vi "hostCommander_old2.vi"() -> ()   [LabVIEW 2014]
uses:
  <vilib>/Platform/TimedLoop/XDataNode/timing_clust.ctl
  <vilib>/Platform/TimedLoop/XDataNode/nitl_modes.ctl
  <vilib>/Platform/TimedLoop/XDataNode/wakeup.ctl
  <vilib>/dex/Stream Element Allocation Mode.ctl
  <vilib>/Analysis/1siggen.llb/Riffle Array (I32).vi
  <vilib>/platform/TimedLoop/XDataNode/XDataNode.xnode
  <resource>/objmgr/ni.dex.rc
  <vilib>/Platform/TimedLoop/XDataNode/XDNodeRunTimeDep.lvlib
  <vilib>/Analysis/NI_AALBase.lvlib
panel:
  out "Tab Control":enum32{"Host Commander"}(tab)
  out "reward#":i32=500
  in  "tickRate":u32=1
  in  "displayLength":dbl=10.0
  out "Digital Waveform Graph":digitalwaveform(graph)
  out "CurTrial#":u16
  out "stateMissed":bool
  out "VSmissed":bool
  out "VSbusy":bool=TRUE caption="VS"
  out "stateBusy":bool=TRUE caption="State"
  in  "FilePath":string="D:\\BehData\\"
  in  "FileName":string="debug"
  in  "Save data":bool=TRUE
  in  "Tab Control _2":T1(tab)
  in  "trialKey":i32[](array[numeric])
  in  "left":i32=300
  in  "right":i32=300
  in  "Initializeation Screen":dbl
  in  "Repeat":dbl
  in  "Interleave":bool
  in  "Randominze":bool
  in  "Blank":bool
  in  "Timing":sgl[](array[numeric])=[0.1, 0.2, 0.4, 0.6, 0.8, 1.0]
  in  "Orientation":sgl[](array[numeric])=[0.1, 0.2, 0.4, 0.6, 0.8, 1.0]
  in  "TF":sgl[](array[numeric])=[0.1, 0.2, 0.4, 0.6, 0.8, 1.0]
  in  "VS type":string="lick_reward"
  in  "SF":sgl[](array[numeric])=[0.04, 0.08, 0.16, 0.32, 0.45]
  in  "rtFIFOsize":u32=50
  in  "rtFIFOtimeout":u32
  in  "rtFIFOdataPool":u32=50
  in  "stateMachineCycle_uS":i64=500
  in  "vsFilterPeriod_uS":i32=500 format="%#1.6f"
  in  "lickThreshold_V":fxp<+/-,16,5>=1.0
  in  "vsThreshold_V":fxp<+/-,16,5>
  in  "audioThreshold_V":fxp<+/-,16,5>
  in  "audioFilterPeriod_uS":i32=50000 format="%#1.6f"
  in  "audioOffState_V":fxp<+/-,16,5>
  in  "manualShock":bool
  in  "manualWaterRight":bool
  in  "manualWaterLeft":bool
  in  "lickReward":bool
  in  "allowPunish":bool
  in  "beh type":string="ToneLickReward"
  in  "toneReward":bool=TRUE
  in  "rwdrefPeriod_uS":u32=500000
  in  "rewardPeriod_uS":u32=500000
  in  "waterOn_uS":u32=35000
  in  "timeout_uS":u32
  in  "shockOn_uS":u32
  in  "delay_uS":u32
  out "current state":u16(ring) items=["idle", "vs before", "vs", "vs after", "delay", "tone before", "tone", "tone after", "cycle end", "reward", "reward refractory", "punish", "punish refractory", "timeout", "exit"]
  out "Error 1":string
  out "Error 2":string
  out "Originating IP":string="192.168.137.2"
  out "Incoming data":string="TrlDone 1.000 "
  out "stream counter":u32
  out "Is Connected":bool
  out "Available Elements for Writing":i32
  in  "stream writer buffer size":i32=500
  in  "IP_VS":string="192.168.137.3"
  in  "IP_RT":string="192.168.137.2"
  in  "port_remote":u16=9091
  in  "IP_host":string="192.168.137.1"
  in  "port_local":u16=9090
  in  "IP_broadcast":string="192.168.137.255"
  out "INFO":string="Stop 1.000 "
  out "stop - local":bool=TRUE
  in  "Notes":string="14-4"
  in  "Abort":bool caption="run-stop"
  in  "run-stop":bool
  out "dispTimeout":bool
  out "saveTimeout":bool
  out "CurTrial# (remote)":u16
  in  "totalTrial#":u16=300
  out "CurTime (min)":i32
  in  "ITI_ms":i32=5000
  # "busy"
  # "missed"
  # "trialProbability"
  # "Errors for debugging"
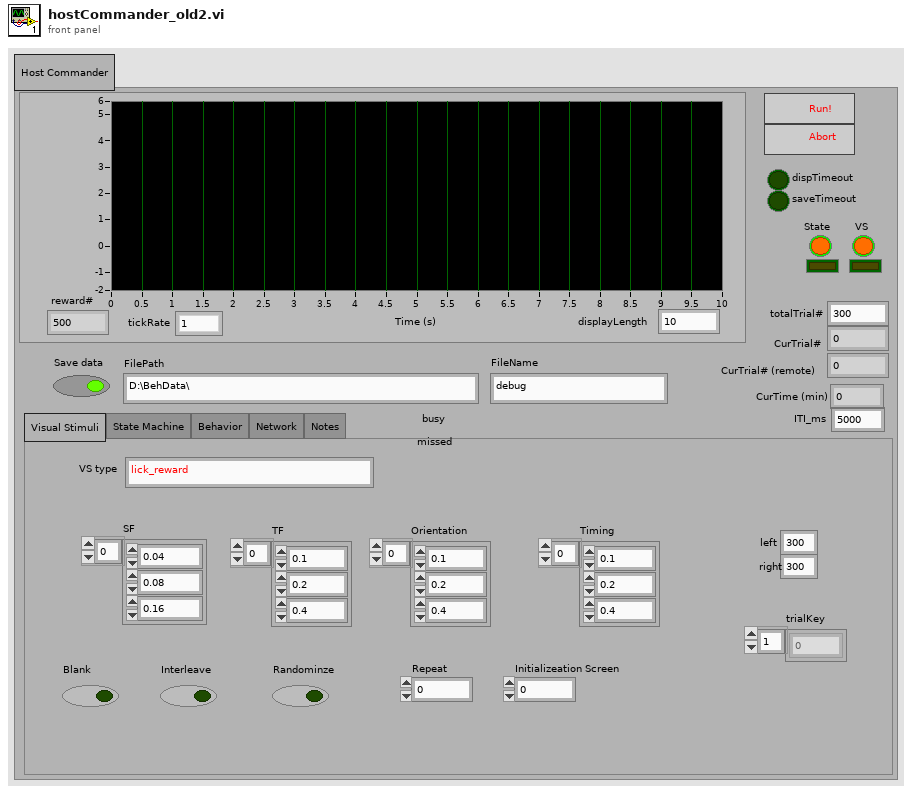
[diagram p1: front panel]
types:
  T1 = enum32{"Visual Stimuli", "State Machine", "Behavior", "Network", "Notes"}
  T2 = enum16{"open", "replace", "create", "open or create", "replace or create", "replace or create with confirmation"}
  T3 = enum16{"big-endian, network order", "native, host order", "little-endian"}
  T4 = typedef "XDNodeRunTimeDep.lvlib/timing_clust.ctl" = cluster{"Expected End [f-1]":u64, "Actual End [f-1]":u64, "Finished Late? [f-1]":bool, "Expected End [i-1]":u64, "Actual End [i-1]":u64, "Finished Late? [i-1]":bool, "Expected Start [i]":u64, "Actual Start [i]":u64, "Expected Start [f]":u64, "Actual Start [f]":u64, "Source Name":string, "Structure Name":string, "Period":i64, "Deadline":i64, "Offset":i64, "Start":i64, "Priority":i32, "Timeout":i32, "Mode":T5, "Wakeup Reason":T6, "Error":errorcluster, "Source Type":string, "Secondary Source Type":string, "Global End Time":u64, "Global Start Time":u64, "Frame Duration":u64, "Iteration Duration":u64, "Assigned CPU":i32, "I/O Scan Engine Mode":u32}
  T5 = typedef "XDNodeRunTimeDep.lvlib/nitl_modes.ctl" = enum32{"No Change", "Process missed periods, maintain original phase", "Discard missed periods, maintain original phase", "Process missed periods, ignore original phase", "Discard missed periods, ignore original phase"}
  T6 = typedef "XDNodeRunTimeDep.lvlib/wakeup.ctl" = enum32{"Normal", "Aborted", "Asynchronous wakeup", "Timing source error", "Timed loop error", "Timeout"}
  T7 = typedef "Stream Element Allocation Mode.ctl" = u32
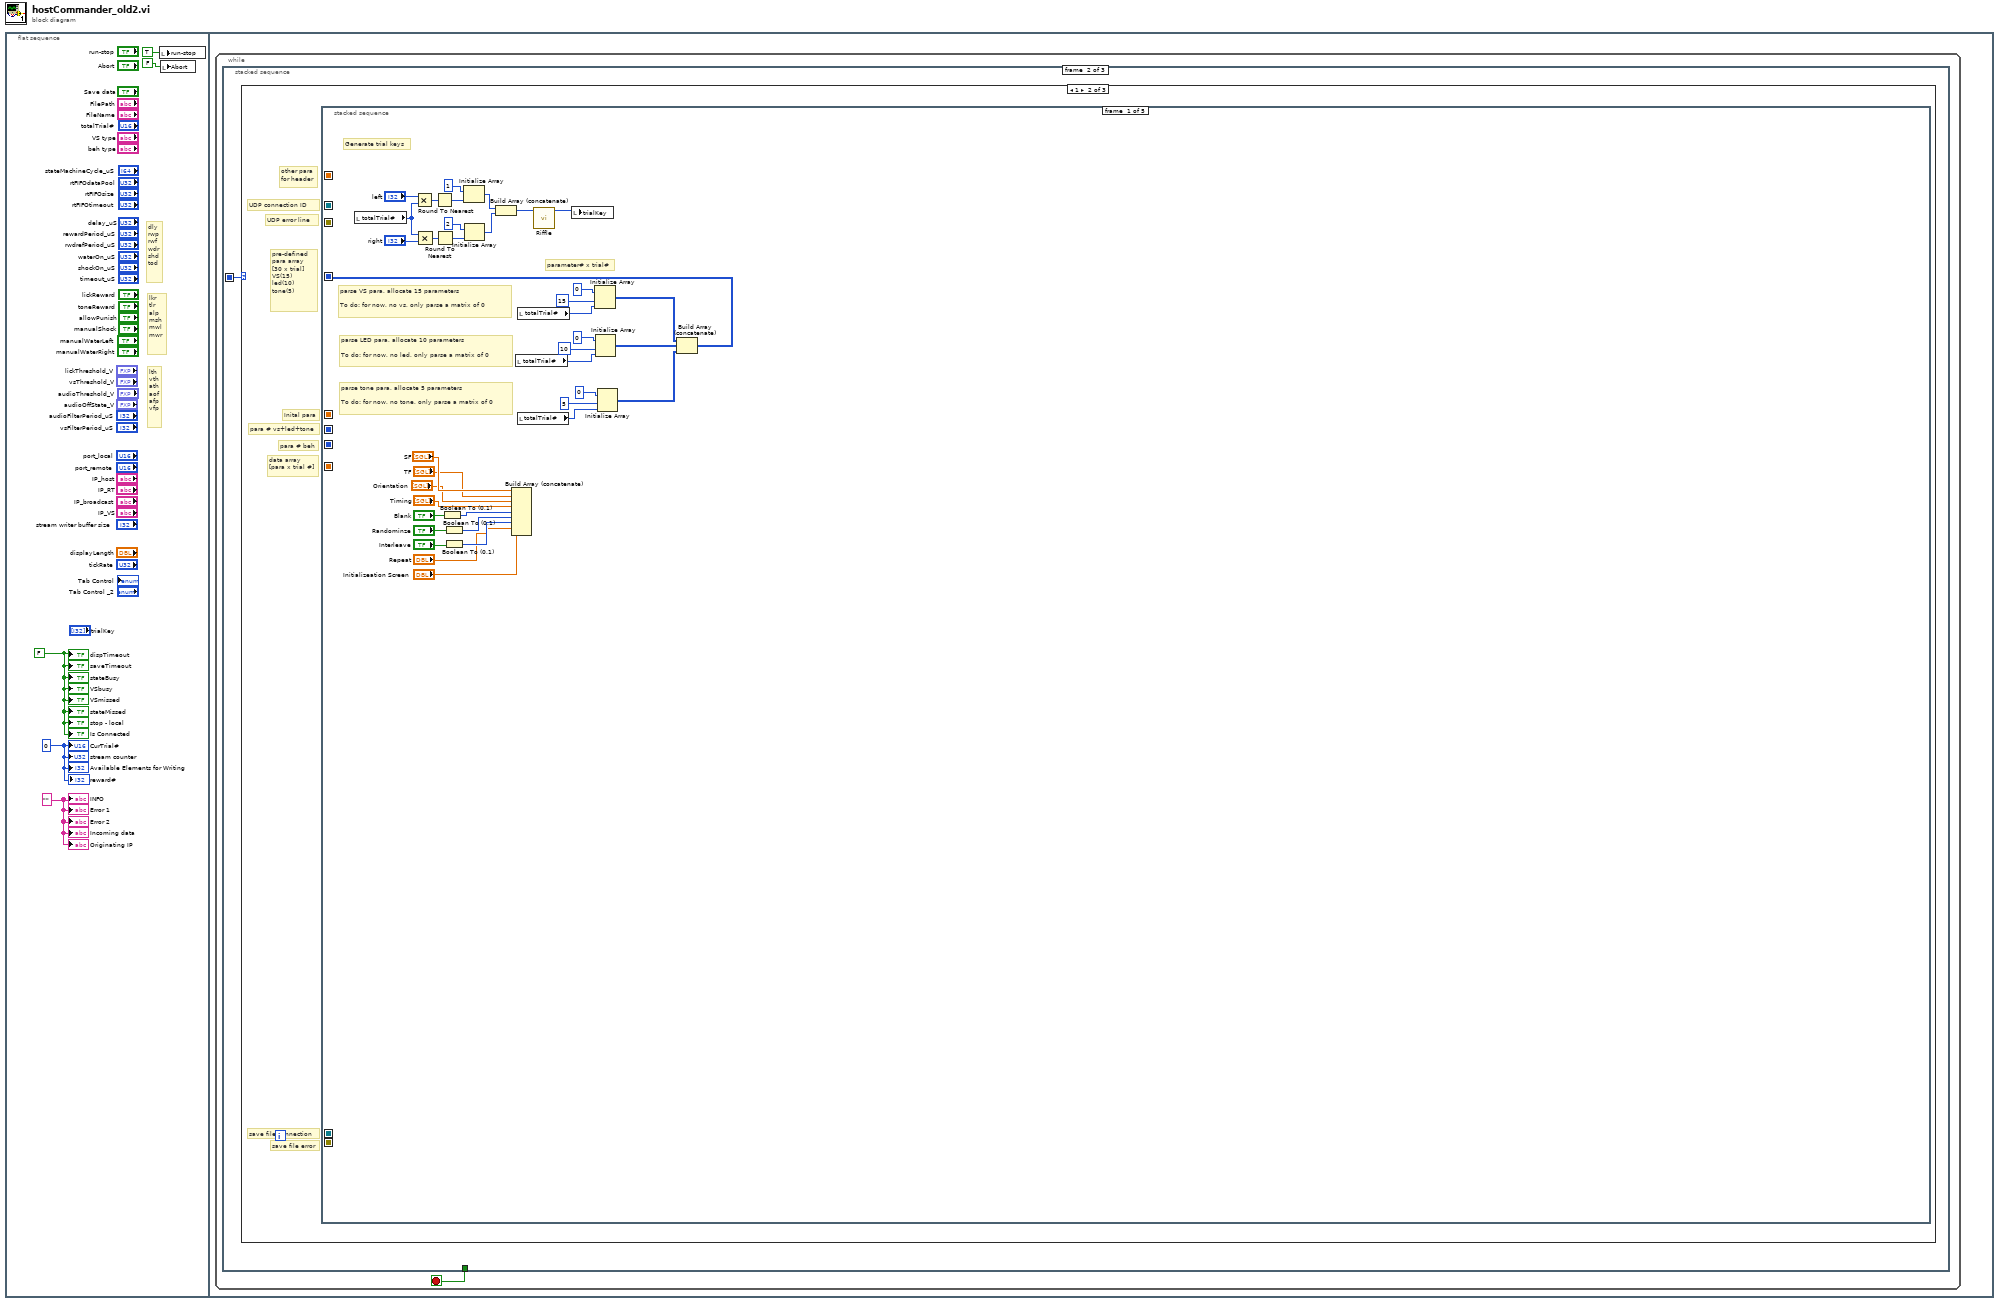
[diagram p0: block diagram]
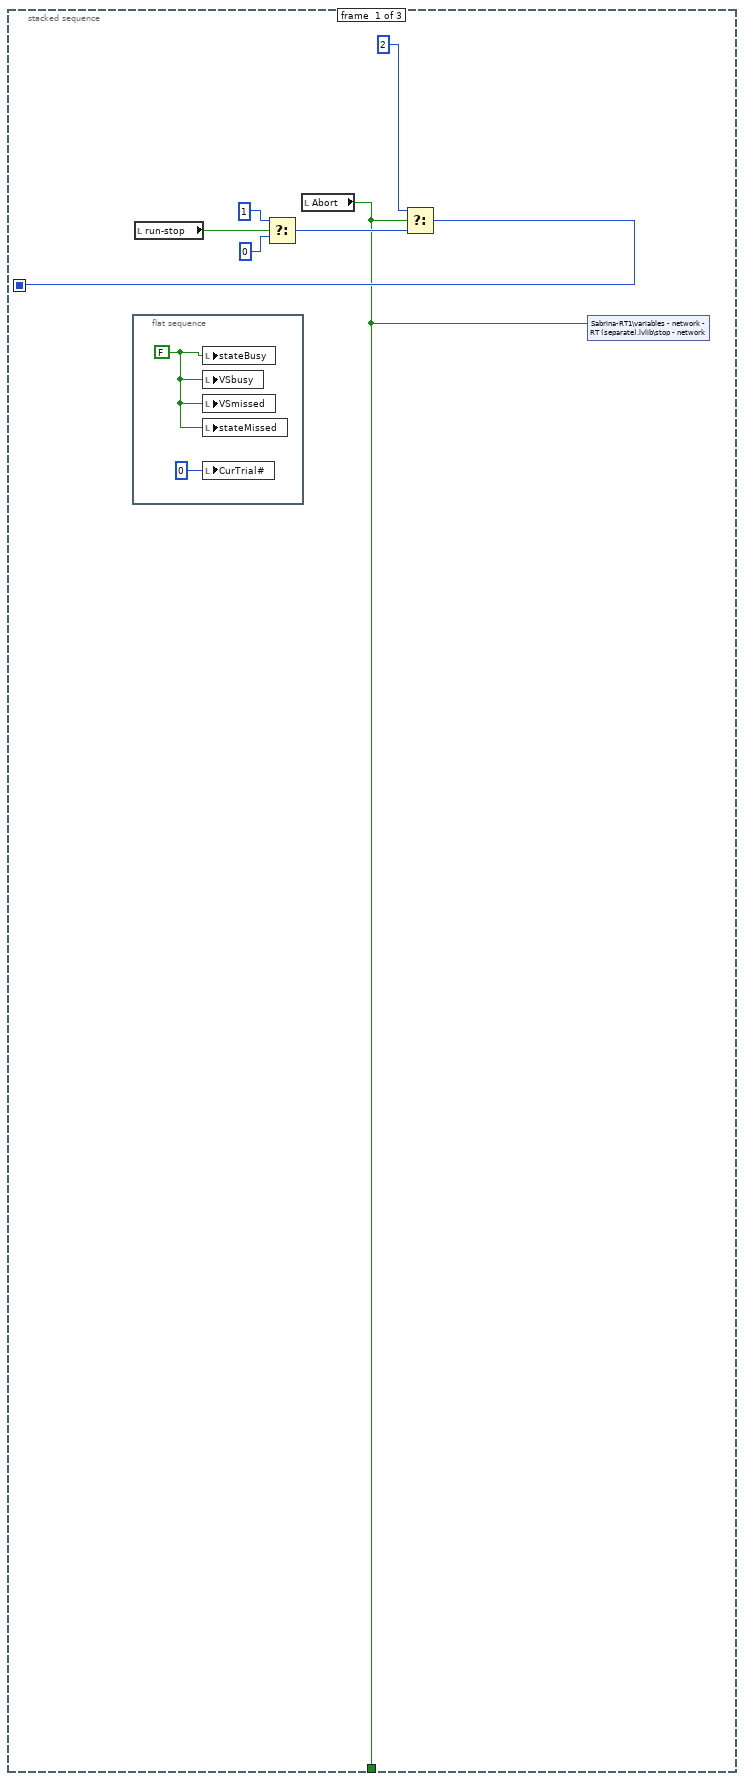
[diagram p2: hidden frame]
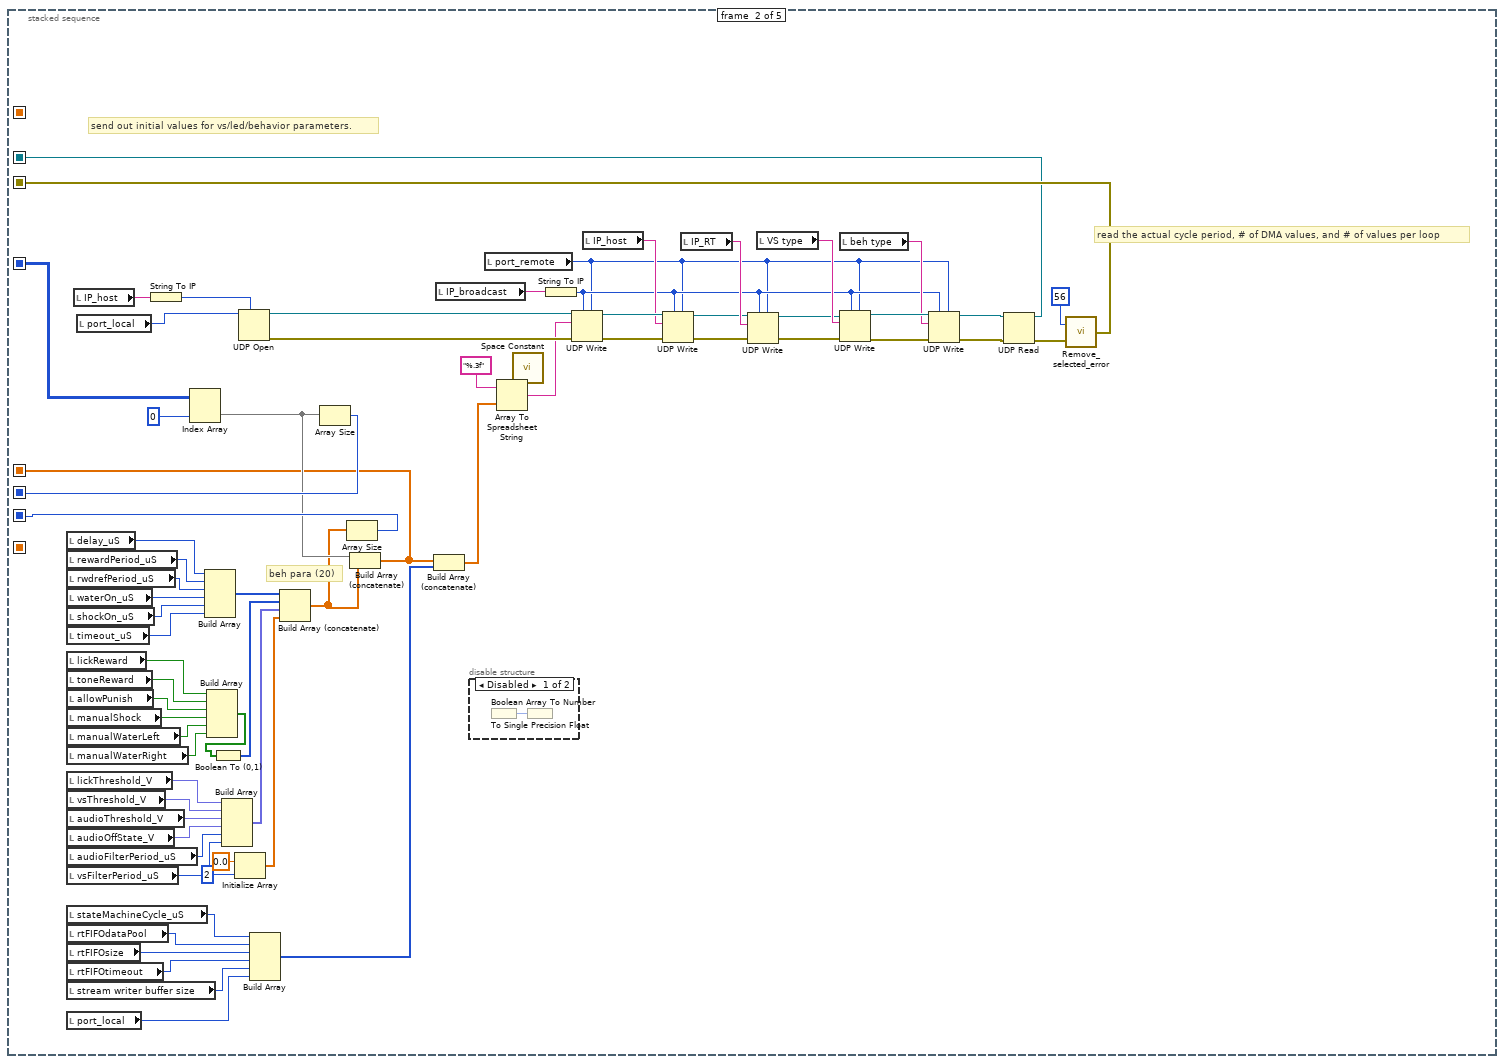
[diagram p4: hidden frame]
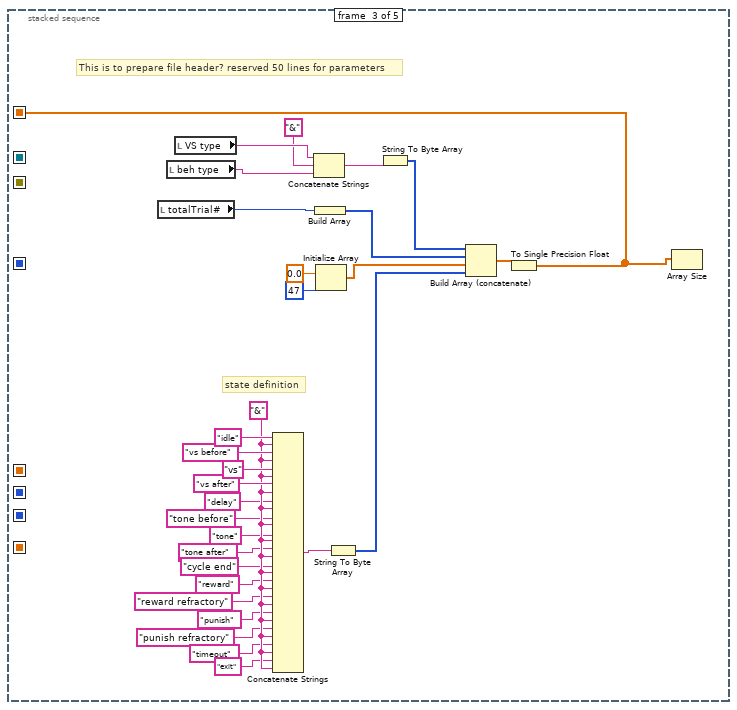
[diagram p6: hidden frame]
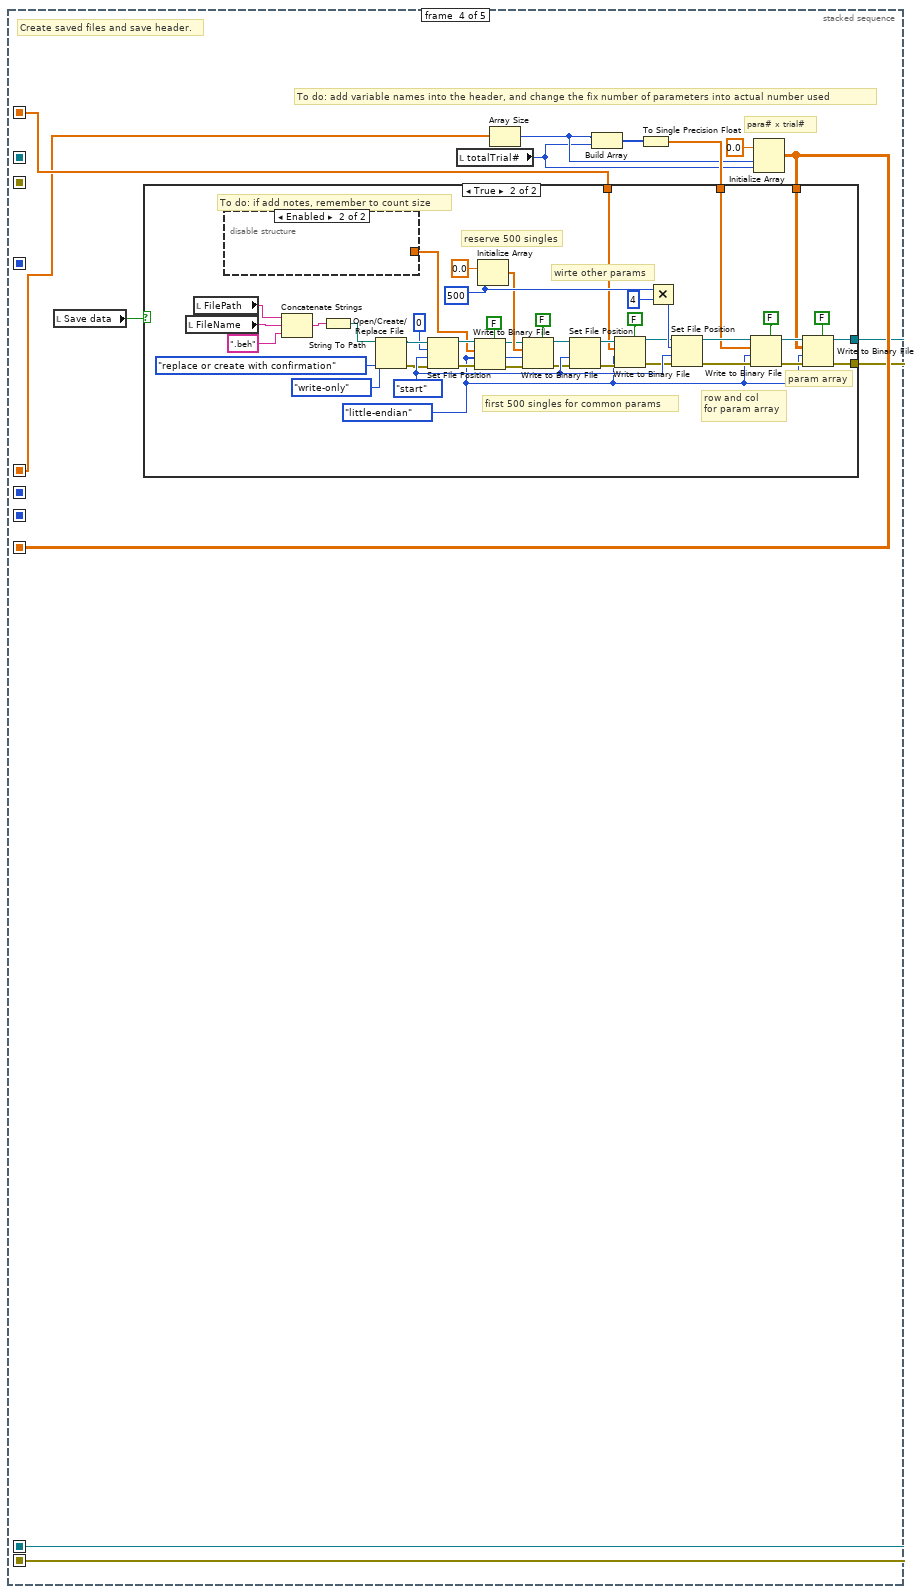
[diagram p7: hidden frame]
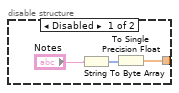
[diagram p9: hidden frame]
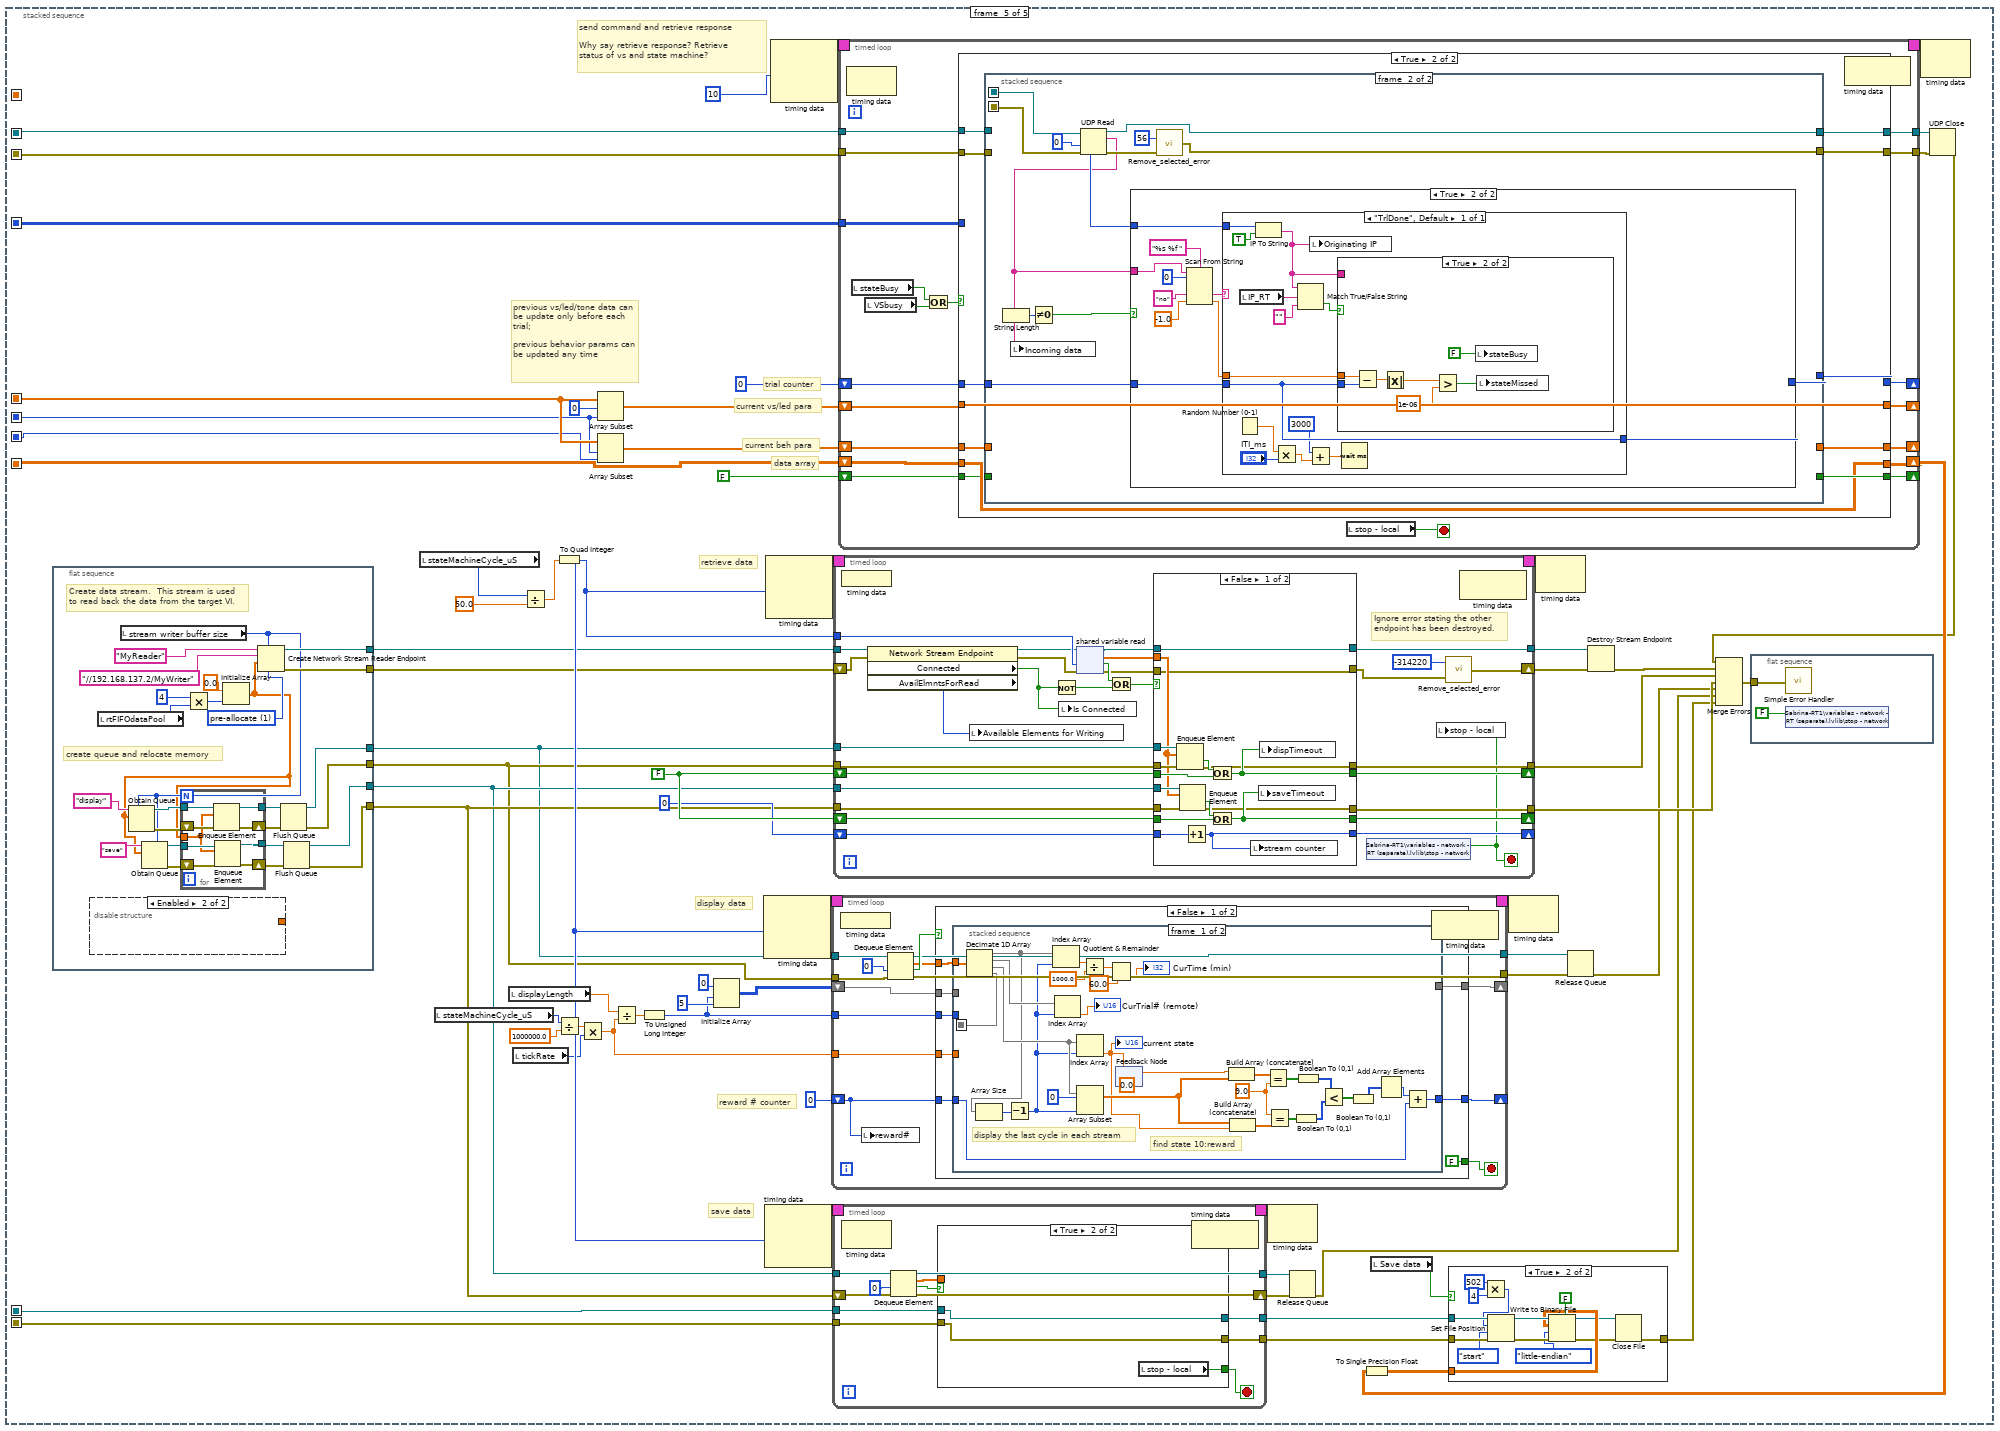
[diagram p10: hidden frame]
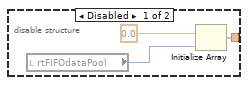
[diagram p11: hidden frame]
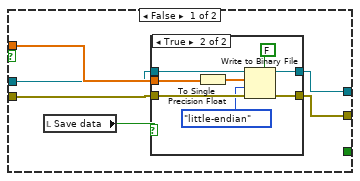
[diagram p12: hidden frame]
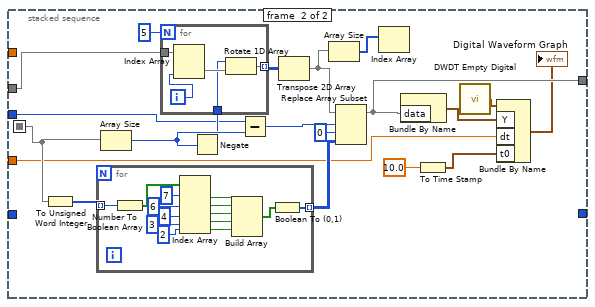
[diagram p14: hidden frame]
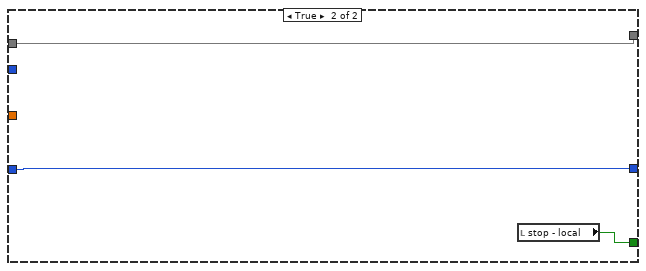
[diagram p15: hidden frame]
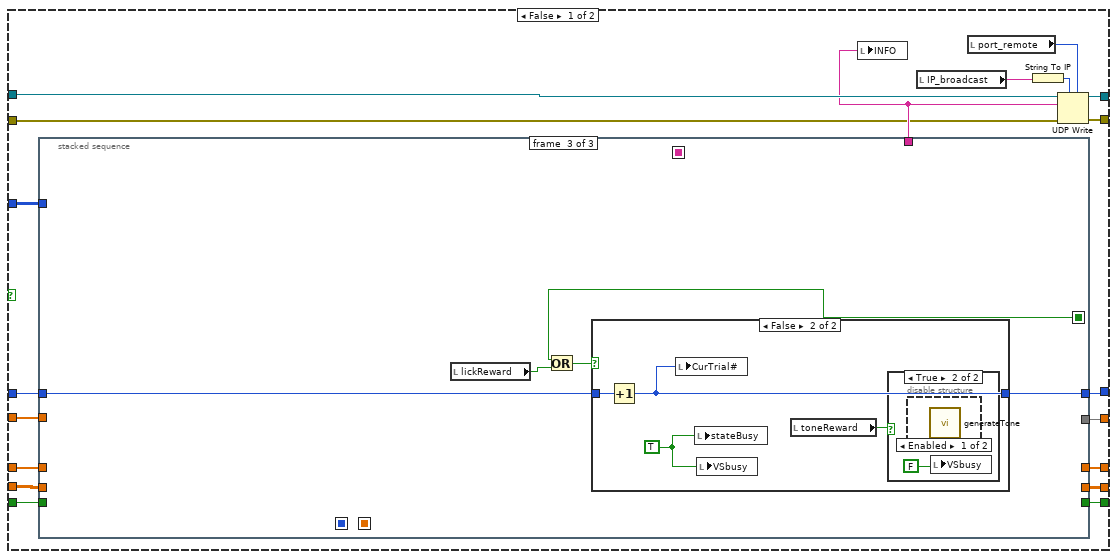
[diagram p17: hidden frame]
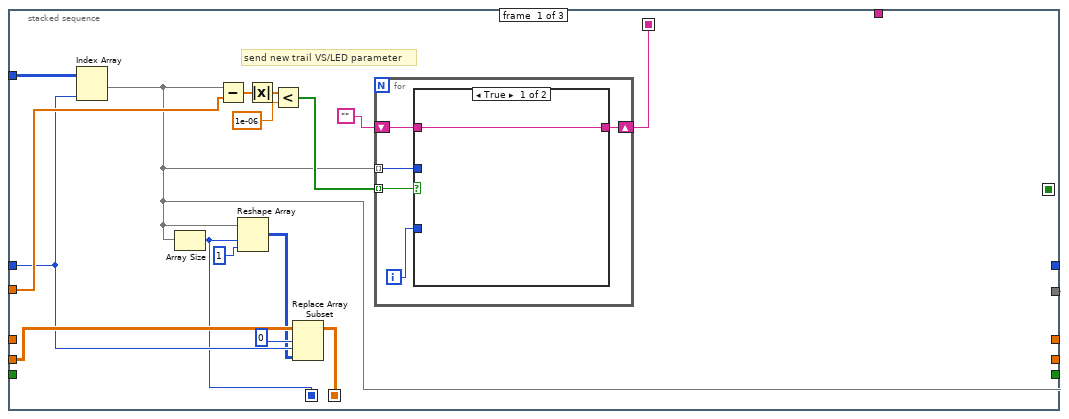
[diagram p18: hidden frame]
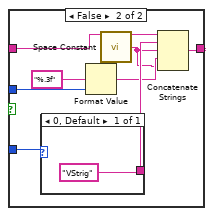
[diagram p19: hidden frame]
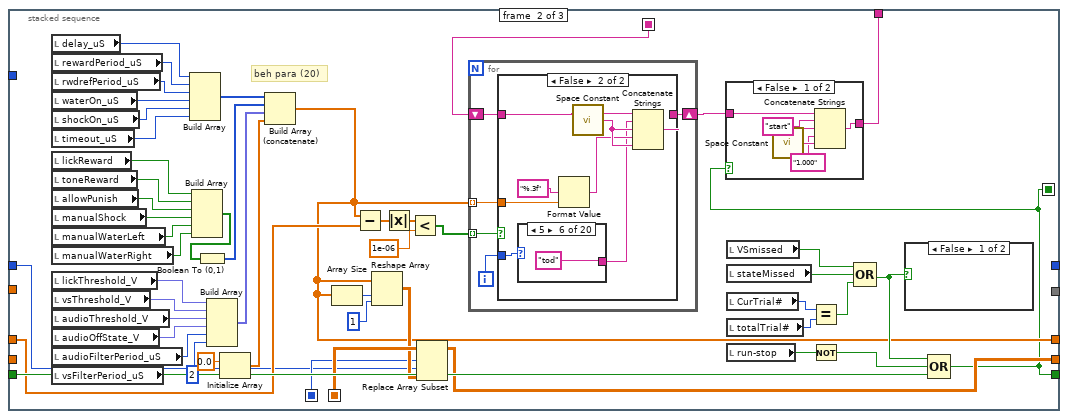
[diagram p20: hidden frame]
diagram:
  n1 = flat-sequence {
    frame #0 {
      w2 = ""
      w1 = 0
      w3 = FALSE
      # "lth\nvth\nath\naof\nafp\nvfp"
      # "dly\nrwp\nrwf\nwdr\nshd\ntod"
      # "lkr\ntlr\nalp\nmsh\nmwl\nmwr"
      n2 = local write "run-stop"(TRUE) -> ()
      n3 = local write "Abort"(FALSE) -> ()
      "dispTimeout" <- w3
      "saveTimeout" <- w3
      "stateBusy" <- w3
      "VSbusy" <- w3
      "VSmissed" <- w3
      "stateMissed" <- w3
      "CurTrial#" <- w1
      "stop - local" <- w3
      "INFO" <- w2
      "Error 2" <- w2
      "Error 1" <- w2
      "Available Elements for Writing" <- w1
      "Is Connected" <- w3
      "stream counter" <- w1
      "Incoming data" <- w2
      "Originating IP" <- w2
      "reward#" <- w1
    }
    frame #1 {
      n4 = while {
        stop <- w6 stop-if-true
        n5 = stacked-sequence {
          seq-local: [w8 _ _] -> [_ w16 _]
          tunnel: [w7 _ _] -> w6
          frame #0 {
            n6 = flat-sequence {
              frame #0 {
                w15 = FALSE
                n7 = local write "stateBusy"(w15) -> ()
                n8 = local write "VSbusy"(w15) -> ()
                n9 = local write "VSmissed"(w15) -> ()
                n10 = local write "stateMissed"(w15) -> ()
                n11 = local write "CurTrial#"(0) -> ()
              }
            }
            n12 = local read "run-stop"() -> (w10:bool)
            n13 = Select(t=u8 1, s=w10, f=u8 0) -> (s? t:f=w9:u8)
            n14 = local read "Abort"() -> (w7:bool)
            n15 = Select(t=u8 2, s=w7, f=w9) -> (s? t:f=w8:u8)
            n16 = shared-variable "Sabrina-RT1\\variables - network - RT (separate).lvlib\\stop - network"(w7) -> ()  [unwired: 1 in, 1 out]
          }
          frame #1 {
            n17 = case shown="1" w16 {
              frame 0, Default {
              }
              frame 1 {
                # "para # beh"
                # "save file error"
                # "save file connection"
                # "data array\n[para x trial #]"
                # "other para\nfor header"
                # "UDP error line"
                # "UDP connection ID"
                # "para # vs+led+tone"
                # "Inital para"
                # "pre-defined \npara array\n[30 x trial]\nVS(15)\nled(10)\ntone(5)"
                n18 = stacked-sequence {
                  seq-local: [_ w105 _ _ _] -> [_ _ _ _ w264]
                  seq-local: [_ w102 _ _ _] -> [_ _ _ _ w265]
                  seq-local: [_ w55 _ _ _] -> [_ _ _ w157 w263]
                  seq-local: [_ w69 _ _ _] -> [_ _ _ _ w213]
                  seq-local: [w37 _ _ _ _] -> [_ w106 _ _ w256]
                  seq-local: [_ _ w125 _ _] -> [_ _ _ w161 _]
                  seq-local: [_ _ _ w160 _] -> [_ _ _ _ w255]
                  seq-local: [_ _ _ w159 _] -> [_ _ _ _ w235]
                  seq-local: [_ _ _ w158 _] -> [_ _ _ _ w236]
                  seq-local: [_ w70 _ _ _] -> [_ _ _ _ w215]
                  frame #0 {
                    # "parameter# x trial#"
                    # "parse tone para, allocate 5 parameters \n\nTo do: for now, no tone, only parse a matrix of 0"
                    # "parse LED para, allocate 10 parameters \n\nTo do: for now, no led, only parse a matrix of 0"
                    # "parse VS para, allocate 15 parameters \n\nTo do: for now, no vs, only parse a matrix of 0"
                    # "Generate trial keys"
                    n19 = local read "totalTrial#"() -> (w21:u16)
                    n20 = Multiply(x="left", y=w21) -> (x*y=w28:i32)
                    n21 = Multiply(x=w21, y="right") -> (x*y=w23:i32)
                    n22 = Round To Nearest(number=w28) -> (nearest integer value=w26:i32)
                    n23 = Round To Nearest(number=w23) -> (nearest integer value=w25:i32)
                    n24 = Boolean To (0,1)(Boolean="Blank") -> (0, 1=w49:i16)
                    n25 = Boolean To (0,1)(Boolean="Interleave") -> (0, 1=w44:i16)
                    n26 = Boolean To (0,1)(Boolean="Randominze") -> (0, 1=w48:i16)
                    n27 = Initialize Array(1, w26) -> (w20:i32[])
                    n28 = Initialize Array(2, w25) -> (w19:i32[])
                    n29 = Build Array (concatenate)(w20, w19) -> (w18:i32[])
                    n30 = Build Array (concatenate)("SF", "TF", "Orientation", "Timing", w49, w48, w44, "Repeat", "Initializeation Screen") -> ()  [unwired: 1 out]
                    n31 = local read "totalTrial#"() -> (w35:u16)
                    n32 = local read "totalTrial#"() -> (w34:u16)
                    n33 = local read "totalTrial#"() -> (w36:u16)
                    n34 = call-poly <vilib>:"Riffle.vi"("X"=w18) -> ("Riffled {X}"=w17:i32[])  [unwired: 8 in, 2 out]
                    n35 = local write "trialKey"(w17) -> ()
                    n36 = Initialize Array(0, 15, w36) -> (w40:i32[][])
                    n37 = Initialize Array(0, 10, w35) -> (w39:i32[][])
                    n38 = Initialize Array(0, 5, w34) -> (w38:i32[][])
                    n39 = Build Array (concatenate)(w40, w39, w38) -> (w37:i32[][])
                  }
                  frame #1 {
                    # "beh para (20)"
                    # "read the actual cycle period, # of DMA values, and # of values per loop"
                    # "send out initial values for vs/led/behavior parameters."
                    n40 = local read "delay_uS"() -> (w99:u32)
                    n41 = local read "rewardPeriod_uS"() -> (w98:u32)
                    n42 = local read "rwdrefPeriod_uS"() -> (w97:u32)
                    n43 = local read "waterOn_uS"() -> (w96:u32)
                    n44 = local read "shockOn_uS"() -> (w95:u32)
                    n45 = local read "timeout_uS"() -> (w94:u32)
                    n46 = local read "lickReward"() -> (w93:bool)
                    n47 = local read "toneReward"() -> (w92:bool)
                    n48 = local read "allowPunish"() -> (w91:bool)
                    n49 = local read "manualShock"() -> (w90:bool)
                    n50 = local read "manualWaterLeft"() -> (w89:bool)
                    n51 = local read "manualWaterRight"() -> (w88:bool)
                    n52 = local read "lickThreshold_V"() -> (w87:fxp<+/-,16,5>)
                    n53 = local read "vsThreshold_V"() -> (w86:fxp<+/-,16,5>)
                    n54 = local read "audioThreshold_V"() -> (w85:fxp<+/-,16,5>)
                    n55 = local read "audioOffState_V"() -> (w82:fxp<+/-,16,5>)
                    n56 = local read "audioFilterPeriod_uS"() -> (w84:i32)
                    n57 = local read "vsFilterPeriod_uS"() -> (w83:i32)
                    n58 = local read "stateMachineCycle_uS"() -> (w81:i64)
                    n59 = local read "rtFIFOdataPool"() -> (w79:u32)
                    n60 = local read "rtFIFOsize"() -> (w78:u32)
                    n61 = local read "rtFIFOtimeout"() -> (w80:u32)
                    n62 = local read "stream writer buffer size"() -> (w77:i32)
                    n63 = local read "port_local"() -> (w68:u16)
                    n64 = local read "IP_host"() -> (w120:string)
                    n65 = local read "port_local"() -> (w118:u16)
                    n66 = String To IP(1:w120) -> (0:w119:u32)
                    n67 = Index Array(array=w106, index (col)=0) -> (element=w57:i32[])  [unwired: 1 in]
                    n68 = Build Array(w99, w98, w97, w96, w95, w94) -> (w76:u32[])
                    n69 = Build Array(w93, w92, w91, w90, w89, w88) -> (w59:bool[])
                    n70 = Boolean To (0,1)(Boolean=w59) -> (0, 1=w58:i16[])
                    n71 = Build Array(w87, w86, w85, w82, w84, w83) -> (w75:fxp<+/-,43,32>[])
                    n72 = Initialize Array(sgl 0.0, 2) -> (w71:sgl[])
                    n73 = UDP Open(7:w119, 11:w118) -> (port=w116:refnum<k16>, 0:w117:errorcluster)  [unwired: 3 in, 1 out]
                    n74 = Build Array(w81, w79, w78, w80, w77, w68) -> (w74:i64[])
                    n75 = Build Array (concatenate)(w76, w58, w75, w71) -> (w56:sgl[])
                    n76 = Array Size(array=w57) -> (size(s)=w69:i32)
                    n77 = Array Size(array=w56) -> (size(s)=w70:i32)
                    n78 = Build Array (concatenate)(w57, w56) -> (w55:sgl[])
                    n79 = Build Array (concatenate)(w55, w74) -> (w107:sgl[])
                    n80 = local read "IP_broadcast"() -> (w121:string)
                    n81 = disable-structure shown="Disabled" {
                      frame Disabled {
                        n82 = Boolean Array To Number() -> (number=w122:u32)  [unwired: 1 in]
                        n83 = To Single Precision Float(number=w122) -> ()  [unwired: 1 out]
                      }
                      frame Enabled {
                      }
                    }
                    n84 = local read "port_remote"() -> (w63:u16)
                    n85 = call <vilib>:"Space Constant.vi"() -> ("String"=w109:string)
                    n86 = Array To Spreadsheet String ("beh para")(delimiter (Tab)=w109, array=w107, 3:"%.3f" ("format string")) -> (spreadsheet string=w108:string)
                    n87 = String To IP(1:w121) -> (0:w64:u32)
                    n88 = UDP Write(address=w64, port or service name=w63, connection ID=w116, data in=w108, 8:w117) -> (error out=w115:errorcluster, 3:w67:refnum<k16>)  [unwired: 1 in]
                    n89 = local read "IP_host"() -> (w66:string)
                    n90 = UDP Write(address=w64, port or service name=w63, connection ID=w67, data in=w66) -> (3:w62:refnum<k16>)  [unwired: 2 in, 1 out]
                    n91 = local read "IP_RT"() -> (w65:string)
                    n92 = UDP Write(address=w64, port or service name=w63, connection ID=w62, data in=w65) -> (3:w61:refnum<k16>)  [unwired: 2 in, 1 out]
                    n93 = local read "VS type"() -> (w114:string)
                    n94 = local read "beh type"() -> (w111:string)
                    n95 = UDP Write(address=w64, port or service name=w63, connection ID=w61, data in=w114, 8:w115) -> (error out=w113:errorcluster, 3:w112:refnum<k16>)  [unwired: 1 in]
                    n96 = UDP Write(address=w64, port or service name=w63, connection ID=w112, data in=w111, 8:w113) -> (error out=w103:errorcluster, 3:w104:refnum<k16>)  [unwired: 1 in]
                    n97 = UDP Read(connection ID=w104, 8:w103) -> (error out=w101:errorcluster, 3:w102:refnum<k16>)  [unwired: 2 in, 3 out]
                    n98 = call "Remove_selected_error.vi"("error in (no error)"=w101, "errorCode"=56) -> ("error out"=w105:errorcluster)
                  }
                  frame #2 {
                    w137 = "&" ("string")
                    # "state definition"
                    # "This is to prepare file header? reserved 50 lines for parameters"
                    n99 = local read "totalTrial#"() -> (w145:u16)
                    n100 = local read "beh type"() -> (w123:string)
                    n101 = local read "VS type"() -> (w140:string)
                    n102 = Concatenate Strings("idle", w137, "vs before", w137, "vs", w137, "vs after", w137, "delay", w137, "tone before", w137, "tone", w137, "tone after", w137, "cycle end", w137, "reward", w137, "reward refractory", w137, "punish", w137, "punish refractory", w137, "timeout", w137, "exit", w137) -> (w150:string)
                    n103 = Concatenate Strings(w140, "&" ("string"), w123) -> (w139:string)
                    n104 = Build Array(w145) -> (w144:u16[])
                    n105 = Initialize Array(sgl 0.0 ("element"), 47 ("dimension size")) -> (w143:sgl[])
                    n106 = String To Byte Array(string=w150) -> (unsigned byte array=w142:u8[])
                    n107 = String To Byte Array(string=w139) -> (unsigned byte array=w138:u8[])
                    n108 = Build Array (concatenate)(w138, w144, w143, w142) -> (w141:sgl[])
                    n109 = To Single Precision Float(number=w141) -> (single precision float=w125:sgl[])
                    n110 = Array Size(array=w125) -> ()  [unwired: 1 out]
                  }
                  frame #3 {
                    # "To do: add variable names into the header, and change the fix number of parameters into actual number used"
                    # "para# x trial#"
                    # "Create saved files and save header."
                    n111 = local read "Save data"() -> (w163:bool)
                    n112 = local read "totalTrial#"() -> (w153:u16)
                    n113 = Array Size(array=w157) -> (size(s)=w154:i32)
                    n114 = Build Array(w154, w153) -> (w156:i32[])
                    n115 = To Single Precision Float(number=w156) -> (single precision float=w155:sgl[])
                    n116 = Initialize Array(sgl 0.0 ("element"), w154, w153) -> (w160:sgl[][])
                    n117 = case shown="True" w163 {
                      tunnel: w155 -> [_ w180]
                      tunnel: w161 -> [_ w164]
                      tunnel: w160 -> [_ w179]
                      tunnel: [_ w177] -> w158
                      tunnel: [_ w178] -> w159
                      frame False {
                      }
                      frame True {
                        w198 = 500 ("dimension size")
                        w171 = T3."little-endian" ("byte order (0:big-endian, network order)")
                        w199 = enum16{"start", "end", "current"}."start" ("from (0:start)")
                        # "To do: if add notes, remember to count size"
                        # "param array"
                        # "row and col\nfor param array"
                        # "first 500 singles for common params"
                        # "reserve 500 singles"
                        # "wirte other params"
                        n118 = local read "FileName"() -> (w166:string)
                        n119 = local read "FilePath"() -> (w169:string)
                        n120 = disable-structure shown="Enabled" {
                          disable-tunnel: [w206 _] -> w170
                          frame Disabled {
                            n121 = String To Byte Array(string="Notes") -> (unsigned byte array=w207:u8[])
                            n122 = To Single Precision Float(number=w207) -> (single precision float=w206:sgl[])
                          }
                          frame Enabled {
                          }
                        }
                        n123 = Concatenate Strings(w169, w166, ".beh" ("string")) -> (w168:string)
                        n124 = String To Path(string=w168) -> (path=w167:path)
                        n125 = Open/Create/Replace File(file path (use dialog)=w167, operation (0:open)=T2."replace or create with confirmation", access (0:read/write)=enum16{"read/write", "read-only", "write-only"}."write-only") -> (refnum out=w184:refnum<file>, error out=w185:errorcluster)  [unwired: 3 in, 1 out]
                        n126 = Set File Position(offset (in bytes) (0)=i64 0, refnum=w184, from (0:start)=w199, error in=w185) -> (refnum out=w175:refnum<file>, error out=w173:errorcluster)
                        n127 = Write to Binary File(file (use dialog)=w175, data=w170, error in=w173, 5:FALSE ("prepend array or string size? (T)"), 9:w171) -> (refnum out=w174:refnum<file>, error out=w172:errorcluster)  [unwired: 1 in, 1 out]
                        n128 = Initialize Array(sgl 0.0 ("element"), w198) -> (w188:sgl[])
                        n129 = Write to Binary File(file (use dialog)=w174, data=w188, error in=w172, 5:FALSE ("prepend array or string size? (T)"), 9:w171) -> (refnum out=w190:refnum<file>, error out=w191:errorcluster)  [unwired: 1 in, 1 out]
                        n130 = Set File Position(refnum=w190, from (0:start)=w199, error in=w191) -> (refnum out=w192:refnum<file>, error out=w193:errorcluster)  [unwired: 1 in]
                        n131 = Write to Binary File(file (use dialog)=w192, data=w164, error in=w193, 5:FALSE ("prepend array or string size? (T)"), 9:w171) -> (refnum out=w194:refnum<file>, error out=w195:errorcluster)  [unwired: 1 in, 1 out]
                        n132 = Multiply(x=w198, y=4) -> (x*y=w196:i32)
                        n133 = Set File Position(offset (in bytes) (0)=w196, refnum=w194, from (0:start)=w199, error in=w195) -> (refnum out=w201:refnum<file>, error out=w202:errorcluster)
                        n134 = Write to Binary File(file (use dialog)=w201, data=w180, error in=w202, 5:FALSE ("prepend array or string size? (T)"), 9:w171) -> (refnum out=w203:refnum<file>, error out=w204:errorcluster)  [unwired: 1 in, 1 out]
                        n135 = Write to Binary File(file (use dialog)=w203, data=w179, error in=w204, 5:FALSE ("prepend array or string size? (T)"), 9:w171) -> (refnum out=w177:refnum<file>, error out=w178:errorcluster)  [unwired: 1 in, 1 out]
                      }
                    }
                  }
                  frame #4 {
                    w270 = FALSE
                    # "reward # counter"
                    # "save data"
                    # "data array"
                    # "current beh para"
                    # "current vs/led para"
                    # "trial counter"
                    # "previous vs/led/tone data can be update only before each trial;\n\nprevious behavior params can be updated any time"
                    # "display data"
                    # "retrieve data"
                    # "send command and retrieve response\n\nWhy say retrieve response? Retrieve\nstatus of vs and state machine?"
                    n136 = flat-sequence {
                      tunnel: [w297] -> w221
                      tunnel: [w296] -> w220
                      tunnel: [w285] -> w219
                      tunnel: [w284] -> w218
                      tunnel: [w283] -> w217
                      tunnel: [w282] -> w216
                      frame #0 {
                        w299 = T7 1 items=["allocate as needed", "pre-allocate"] ("element allocation mode")
                        # "create queue and relocate memory"
                        # "Create data stream.  This stream is used\nto read back the data from the target VI."
                        n137 = disable-structure shown="Enabled" {
                          disable-tunnel: [w302 _] -> _
                          frame Disabled {
                            n138 = local read "rtFIFOdataPool"() -> (w303:u32)
                            n139 = Initialize Array(sgl 0.0, w303) -> (w302:sgl[])
                          }
                          frame Enabled {
                          }
                        }
                        n140 = local read "rtFIFOdataPool"() -> (w278:u32)
                        n141 = local read "stream writer buffer size"() -> (w281:i32)
                        n142 = Multiply(x=4, y=w278) -> (x*y=w277:u32)
                        n143 = Initialize Array(sgl 0.0, w277) -> (w280:sgl[])
                        n144 = Obtain Queue(max queue size (-1, unlimited)=w281, name (unnamed)="display", element data type=w280) -> (queue out=w288:refnum<queue>, error out=w289:errorcluster)  [unwired: 2 in, 1 out]
                        n145 = Obtain Queue(max queue size (-1, unlimited)=w281, name (unnamed)="save", element data type=w280) -> (queue out=w290:refnum<queue>, error out=w291:errorcluster)  [unwired: 2 in, 1 out]
                        n146 = for {
                          N: w281 -> [_]
                          tunnel: w288 -> [w313]
                          tunnel: [w312] -> w294
                          shift-right: [w310] -> w295
                          shift-left: w289 -> [w311]
                          shift-right: [w306] -> w293
                          shift-left: w291 -> [w307]
                          tunnel: w290 -> [w309]
                          tunnel: [w308] -> w292
                          tunnel: w280 -> [w305]
                          n147 = Enqueue Element(queue=w313, element=w305, error in (no error)=w311) -> (queue out=w312:refnum<queue>, error out=w310:errorcluster)  [unwired: 1 in, 1 out]
                          n148 = Enqueue Element(queue=w309, element=w305, error in (no error)=w307) -> (queue out=w308:refnum<queue>, error out=w306:errorcluster)  [unwired: 1 in, 1 out]
                        }
                        n149 = Create Network Stream Reader Endpoint(6:w299, 7:w281, 9:w280, 10:"//192.168.137.2/MyWriter" ("reader name"), 11:"MyReader" ("reader name")) -> (0:w297:errorcluster, 3:w296:refnum<k21>)  [unwired: 2 in]
                        n150 = Flush Queue(queue=w294, error in (no error)=w295) -> (queue out=w282:refnum<queue>, error out=w283:errorcluster)  [unwired: 1 out]
                        n151 = Flush Queue(queue=w292, error in (no error)=w293) -> (queue out=w284:refnum<queue>, error out=w285:errorcluster)  [unwired: 1 out]
                      }
                    }
                    n152 = local read "stateMachineCycle_uS"() -> (w273:i64)
                    n153 = local read "stateMachineCycle_uS"() -> (w249:i64)
                    n154 = local read "displayLength"() -> (w243:dbl)
                    n155 = local read "tickRate"() -> (w211:u32)
                    n156 = Divide(x=w273, y=sgl 50.0) -> (x/y=w272:sgl)
                    n157 = To Quad Integer(1:w272) -> (0:w222:i64)
                    n158 = Divide(x=w249, y=1000000.0) -> (x/y=w212:dbl)
                    n159 = Multiply(x=w212, y=w211) -> (x*y=w210:dbl)
                    n160 = Array Subset(array=w263, index=0, length=w213) -> (w261:sgl[])
                    n161 = Array Subset(array=w263, index=w213, length=w215) -> (w262:sgl[])
                    n162 = Divide(x=w243, y=w210) -> (x/y=w246:dbl)
                    n163 = To Unsigned Long Integer(number=w246) -> (unsigned 32bit integer=w244:u32)
                    n164 = Initialize Array(u8 0, w244, 5 ("dimension size")) -> (w245:u8[][])
                    n165 = node-c288(w222) -> (w242:T4)  [unwired: 2 in]
                    n166 = node-c288(w222) -> (w240:T4)  [unwired: 2 in]
                    n167 = node-c288(w222) -> (w276:T4)  [unwired: 2 in]
                    n168 = node-c288(10) -> (w267:T4)  [unwired: 2 in]
                    n169 = timed-loop {
                      tunnel: w216 -> [w366]
                      tunnel: w217 -> [w365]
                      shift-right: [w362] -> _
                      shift-left: u32 0 -> [w353]
                      shift-right: [w359] -> _
                      shift-left: w245 -> [w361]
                      tunnel: w244 -> [w360]
                      timing: w242 -> [_]
                      timing-out: [_] -> w241
                      tunnel: [w356] -> w232
                      tunnel: [w355] -> w231
                      tunnel: w210 -> [w354]
                      stop <- w358 stop-if-true
                      n170 = node-c288() -> ()  [unwired: 1 in]
                      n171 = local write "reward#"(w353) -> ()
                      n172 = Dequeue Element(queue=w366, timeout in ms (-1)=0, error in (no error)=w365) -> (queue out=w356:refnum<queue>, element=w363:sgl[], timed out?=w364:bool, error out=w355:errorcluster)
                      n173 = case shown="False" w364 {
                        tunnel: w363 -> [w376 _]
                        tunnel: w353 -> [w375 w446]
                        tunnel: [w374 w446] -> w362
                        tunnel: w361 -> [w373 w447]
                        tunnel: w360 -> [w372 _]
                        tunnel: [w371 w447] -> w359
                        tunnel: [FALSE w448] -> w358
                        tunnel: w354 -> [w369 _]
                        frame False {
                          n174 = stacked-sequence {
                            seq-local: [w395 _] -> [_ w418]
                            tunnel: w376 -> [w406 _]
                            tunnel: w375 -> [w390 _]
                            tunnel: [w396 _] -> w374
                            tunnel: w373 -> [_ w417]
                            tunnel: w372 -> [_ w409]
                            tunnel: [_ w412] -> w371
                            tunnel: w369 -> [_ w410]
                            frame #0 {
                              w384 = sgl 9.0
                              # "display the last cycle in each stream"
                              # "find state 10:reward"
                              n175 = Decimate 1D Array(w406) -> (w391:sgl[], w393:sgl[], w392:sgl[], w395:sgl[])
                              n176 = Array Size(array=w391) -> (size(s)=w389:i32)
                              n177 = Decrement(x=w389) -> (x-1=w388:i32)
                              n178 = Index Array(array=w391, index=w388) -> (element=w397:sgl)
                              n179 = Index Array(array=w393, index=w388) -> (element=→"CurTrial# (remote)":sgl)
                              n180 = Index Array(array=w392, index=w388) -> (element=w386:sgl)
                              "current state" <- w386
                              n181 = Array Subset(array=w392, index=0, length=w388) -> (w387:sgl[])
                              n182 = Divide(x=w397, y=sgl 1000.0) -> (x/y=w399:sgl)
                              n183 = Quotient & Remainder(x=w399, y=sgl 60.0) -> (floor(x/y)=→"CurTime (min)":sgl)  [unwired: 1 out]
                              n184 = feedback #1(sgl 0.0) -> (w402:sgl)
                              n185 = feedback-in #1(w386) -> ()
                              n186 = Build Array (concatenate)(w402, w387) -> (w385:sgl[])
                              n187 = Build Array (concatenate)(w387, w386) -> (w383:sgl[])
                              n188 = Equal?(x=w385, y=w384) -> (x = y?=w381:bool[])
                              n189 = Equal?(x=w384, y=w383) -> (x = y?=w380:bool[])
                              n190 = Boolean To (0,1)(Boolean=w380) -> (0, 1=w378:i16[])
                              n191 = Boolean To (0,1)(Boolean=w381) -> (0, 1=w379:i16[])
                              n192 = Less?(x=w379, y=w378) -> (x < y?=w382:bool[])
                              n193 = Boolean To (0,1)(Boolean=w382) -> (0, 1=w404:i16[])
                              n194 = Add Array Elements(numeric array=w404) -> (sum=w405:i16)
                              n195 = Add(x=w405, y=w390) -> (x+y=w396:u32)
                            }
                            frame #1 {
                              n196 = To Unsigned Word Integer(number=w418) -> (unsigned 16bit integer=w419:u16[])
                              n197 = for {
                                tunnel: w419 -> [w445] mode=indexing
                                tunnel: [w432] -> w421 mode=indexing
                                n198 = Number To Boolean Array(number=w445) -> (Boolean array=w444:bool[])
                                n199 = Index Array(array=w444, index #1=7, index #2=6, index #3=4, index #4=3, index #5=2) -> (element #1=w443:bool, element #2=w442:bool, element #3=w441:bool, element #4=w440:bool, element #5=w439:bool)
                                n200 = Build Array(w443, w442, w441, w440, w439) -> (w433:bool[])
                                n201 = Boolean To (0,1)(Boolean=w433) -> (0, 1=w432:i16[])
                              }
                              n202 = Array Size(array=w418) -> (size(s)=w426:i32)
                              n203 = Negate(x=w426) -> (-x=w424:i32)
                              n204 = for {
                                N: 5 -> [_]
                                tunnel: w417 -> [w431]
                                tunnel: w424 -> [w428]
                                tunnel: [w427] -> w425 mode=indexing
                                i -> [w430]
                                n205 = Index Array(array=w431, index (col)=w430) -> (element=w429:u8[])  [unwired: 1 in]
                                n206 = Rotate 1D Array(1:w429, 2:w428) -> (0:w427:u8[])
                              }
                              n207 = Subtract(x=w409, y=w426) -> (x-y=w420:u32)
                              n208 = Transpose 2D Array(2D array=w425) -> (transposed array=w407:u8[][])
                              n209 = Array Size(array=w407) -> (size(s)=w408:i32[])
                              n210 = Replace Array Subset(array=w407, new element=w421, index (row)=w420, index (col)=0 ("disabled index (col)")) -> (w412:u8[][])
                              n211 = Index Array(array=w408) -> ()  [unwired: 1 in, 1 out]
                              n212 = Bundle By Name ("Build Digital Data")("data"=w412) -> (w414:digitaldata)  [unwired: 1 in]
                              n213 = To Time Stamp(1:10.0 ("number")) -> (0:w416:timestamp)
                              n214 = call <vilib>:"DWDT Empty Digital.vi"() -> ("digital waveform out"=w413:digitalwaveform)  [unwired: 5 in]
                              n215 = Bundle By Name ("Build Waveform")(cluster=w413, "Y"=w414, "dt"=w410, "t0"=w416) -> (→"Digital Waveform Graph":digitalwaveform)
                            }
                          }
                        }
                        frame True {
                          n216 = local read "stop - local"() -> (w448:bool)
                        }
                      }
                      n217 = node-c288() -> ()  [unwired: 1 in, 1 out]
                    }
                    n218 = timed-loop {
                      timing: w240 -> [_]
                      timing-out: [_] -> w239
                      tunnel: w218 -> [w326]
                      tunnel: [w322] -> w238
                      shift-right: [w321] -> w237
                      shift-left: w219 -> [w325]
                      tunnel: w236 -> [w320]
                      tunnel: w235 -> [w319]
                      tunnel: [w318] -> w234
                      tunnel: [w317] -> w233
                      stop <- w316 stop-if-true
                      n219 = node-c288() -> ()  [unwired: 1 in, 1 out]
                      n220 = Dequeue Element(queue=w326, timeout in ms (-1)=0, error in (no error)=w325) -> (queue out=w322:refnum<queue>, element=w323:sgl[], timed out?=w324:bool, error out=w321:errorcluster)
                      n221 = case shown="True" w324 {
                        tunnel: w323 -> [w332 _]
                        tunnel: w320 -> [w331 w346]
                        tunnel: w319 -> [w330 w345]
                        tunnel: [w329 w346] -> w318
                        tunnel: [w328 w345] -> w317
                        tunnel: [_ w344] -> w316
                        frame False {
                          n222 = local read "Save data"() -> (w333:bool)
                          n223 = case shown="True" w333 {
                            tunnel: w331 -> [w334 w343]
                            tunnel: w330 -> [w335 w342]
                            tunnel: w332 -> [_ w337]
                            tunnel: [w335 w339] -> w328
                            tunnel: [w334 w338] -> w329
                            frame False {
                            }
                            frame True {
                              n224 = To Single Precision Float(number=w337) -> (single precision float=w336:sgl[])
                              n225 = Write to Binary File(file (use dialog)=w343, data=w336, error in=w342, 5:FALSE ("prepend array or string size? (T)"), 9:T3."little-endian" ("byte order (0:big-endian, network order)")) -> (refnum out=w338:refnum<file>, error out=w339:errorcluster)  [unwired: 1 in, 1 out]
                            }
                          }
                        }
                        frame True {
                          n226 = local read "stop - local"() -> (w344:bool)
                        }
                      }
                      n227 = node-c288() -> ()  [unwired: 1 in, 1 out]
                    }
                    n228 = timed-loop {
                      timing: w276 -> [_]
                      timing-out: [_] -> w275
                      tunnel: w222 -> [w814]
                      tunnel: [w832] -> w271
                      tunnel: w220 -> [w831]
                      tunnel: w216 -> [w830]
                      tunnel: w217 -> [w829]
                      tunnel: w218 -> [w828]
                      tunnel: w219 -> [w827]
                      shift-right: [w825] -> _
                      shift-left: w270 -> [w826]
                      shift-right: [w823] -> _
                      shift-left: w270 -> [w824]
                      tunnel: [w822] -> w224
                      tunnel: [w821] -> w228
                      shift-right: [w819] -> _
                      shift-left: u32 0 -> [w820]
                      shift-right: [w811] -> w268
                      shift-left: w221 -> [w812]
                      stop <- w808 stop-if-true
                      # "Ignore error stating the other\nendpoint has been destroyed."
                      n229 = node-c288() -> ()  [unwired: 1 in]
                      n230 = property class="Network Stream Endpoint"(reference=w831, error in=w812) -> (reference out=w810:refnum<k21>, error out=w815:errorcluster, "Connected"=w835:bool, "AvailElmntsForRead"=w836:i32)
                      n231 = local write "Available Elements for Writing"(w836) -> ()
                      n232 = Not(x=w835) -> (.not. x?=w834:bool)
                      n233 = local write "Is Connected"(w835) -> ()
                      n234 = shared-variable-read(w810, w815, w814) -> (w817:refnum<k21>, w813:errorcluster, w818:bool, w816:sgl[])
                      n235 = Or(x=w818, y=w834) -> (x .or. y?=w833:bool)
                      n236 = case shown="False" w833 {
                        tunnel: w817 -> [w849 w860]
                        tunnel: [w849 w860] -> w832
                        tunnel: w830 -> [w853 _]
                        tunnel: w829 -> [w851 w857]
                        tunnel: w828 -> [w852 _]
                        tunnel: w827 -> [w850 w856]
                        tunnel: w826 -> [w847 w859]
                        tunnel: [w843 w859] -> w825
                        tunnel: w824 -> [w846 w858]
                        tunnel: [w845 w858] -> w823
                        tunnel: [w842 w857] -> w822
                        tunnel: [w841 w856] -> w821
                        tunnel: w820 -> [w840 w855]
                        tunnel: [w839 w855] -> w819
                        tunnel: w816 -> [w838 _]
                        tunnel: [w837 w854] -> w809
                        tunnel: w813 -> [w837 w854]
                        frame False {
                          n237 = Enqueue Element(queue=w853, element=w838, error in (no error)=w851) -> (timed out?=w848:bool, error out=w842:errorcluster)  [unwired: 1 in, 1 out]
                          n238 = Enqueue Element(queue=w852, element=w838, error in (no error)=w850) -> (timed out?=w844:bool, error out=w841:errorcluster)  [unwired: 1 in, 1 out]
                          n239 = Increment(x=w840) -> (x+1=w839:u32)
                          n240 = Or(x=w848, y=w847) -> (x .or. y?=w843:bool)
                          n241 = Or(x=w844, y=w846) -> (x .or. y?=w845:bool)
                          n242 = local write "stream counter"(w839) -> ()
                          n243 = local write "saveTimeout"(w845) -> ()
                          n244 = local write "dispTimeout"(w843) -> ()
                        }
                        frame True {
                        }
                      }
                      n245 = shared-variable "Sabrina-RT1\\variables - network - RT (separate).lvlib\\stop - network"() -> (w808:bool)  [unwired: 1 in, 1 out]
                      n246 = local write "stop - local"(w808) -> ()
                      n247 = call "Remove_selected_error.vi"("error in (no error)"=w809, "errorCode"=-314220) -> ("error out"=w811:errorcluster)
                      n248 = node-c288() -> ()  [unwired: 1 in, 1 out]
                    }
                    n249 = timed-loop {
                      timing: w267 -> [_]
                      timing-out: [_] -> w266
                      tunnel: w265 -> [w483]
                      tunnel: w264 -> [w482]
                      shift-right: [w480] -> _
                      shift-left: w262 -> [w481]
                      tunnel: [w479] -> w260
                      tunnel: [w478] -> w259
                      shift-right: [w476] -> _
                      shift-left: 0 ("index") -> [w477]
                      shift-right: [w474] -> _
                      shift-left: FALSE -> [w475]
                      tunnel: w256 -> [w473]
                      shift-right: [w471] -> w252
                      shift-left: w255 -> [w472]
                      shift-right: [w469] -> _
                      shift-left: w261 -> [w470]
                      stop <- w468 stop-if-true
                      n250 = node-c288() -> ()  [unwired: 1 in, 1 out]
                      n251 = local read "stateBusy"() -> (w486:bool)
                      n252 = local read "VSbusy"() -> (w485:bool)
                      n253 = Or(x=w486, y=w485) -> (x .or. y?=w484:bool)
                      n254 = case shown="True" w484 {
                        tunnel: w483 -> [w499 w651]
                        tunnel: w482 -> [w492 w650]
                        tunnel: w481 -> [w502 w649]
                        tunnel: [w489 w648] -> w480
                        tunnel: [w498 w647] -> w479
                        tunnel: [w493 w646] -> w478
                        tunnel: w477 -> [w487 w645]
                        tunnel: [w505 w644] -> w476
                        tunnel: w475 -> [w504 w640]
                        tunnel: [w488 w643] -> w474
                        tunnel: w473 -> [w503 _]
                        tunnel: w472 -> [w501 w642]
                        tunnel: [w500 w642] -> w471
                        tunnel: w470 -> [w491 w641]
                        tunnel: [w490 w641] -> w469
                        frame False {
                          n255 = stacked-sequence {
                            seq-local: [w514 _ _] -> [_ w574 _]
                            seq-local: [w507 _ _] -> [_ w543 _]
                            seq-local: [w513 _ _] -> [_ w544 _]
                            seq-local: [_ w537 _] -> [_ _ w631]
                            tunnel: w487 -> [w510 w542 w633]
                            tunnel: [_ _ w632] -> w505
                            tunnel: w504 -> [_ w581 _]
                            tunnel: w503 -> [w521 _ _]
                            tunnel: w502 -> [_ w579 _]
                            tunnel: w501 -> [w515 _ _]
                            tunnel: [_ w572 _] -> w500
                            tunnel: [_ w570 _] -> w495
                            tunnel: w491 -> [w512 _ _]
                            tunnel: [w511 _ _] -> w490
                            tunnel: [_ w545 _] -> w489
                            tunnel: [_ w537 _] -> w488
                            frame #0 {
                              # "send new trail VS/LED parameter"
                              n256 = Index Array(array=w521, index (col)=w510) -> (element=w511:i32[])  [unwired: 1 in]
                              n257 = Array Size(array=w511) -> (size(s)=w507:i32)
                              n258 = Subtract(x=w511, y=w512) -> (x-y=w520:sgl[])
                              n259 = Reshape Array(w511, w507, 1 ("dimension size")) -> (w506:i32[][])
                              n260 = Absolute Value(x=w520) -> (abs(x)=w519:sgl[])
                              n261 = Less?(x=w519, y=1e-06) -> (x < y?=w517:bool[])
                              n262 = Replace Array Subset(array=w515, new element=w506, index (row)=0 ("dimension size"), index (col)=w510) -> (w514:sgl[][])
                              n263 = for {
                                tunnel: w517 -> [w526] mode=indexing
                                shift-right: [w524] -> w513
                                shift-left: "" -> [w525]
                                tunnel: w511 -> [w523] mode=indexing
                                i -> [w522]
                                n264 = case shown="True" w526 {
                                tunnel: w525 -> [w527 w535]
                                tunnel: [w527 w534] -> w524
                                tunnel: w523 -> [_ w529]
                                tunnel: w522 -> [_ w528]
                                frame True {
                                }
                                frame False {
                                n265 = case shown="0, Default" w528 {
                                tunnel: ["VStrig"] -> w533
                                frame 0, Default {
                                }
                                }
                                n266 = Format Value(format string="%.3f", value (0)=w529) -> (output string=w532:string)  [unwired: 1 in]
                                n267 = call <vilib>:"Space Constant.vi"() -> ("String"=w531:string)
                                n268 = Concatenate Strings(w535, w533, w531, w532, w531) -> (w534:string)
                                }
                                }
                              }
                            }
                            frame #1 {
                              # "beh para (20)"
                              n269 = local read "delay_uS"() -> (w568:u32)
                              n270 = local read "rewardPeriod_uS"() -> (w567:u32)
                              n271 = local read "rwdrefPeriod_uS"() -> (w566:u32)
                              n272 = local read "waterOn_uS"() -> (w565:u32)
                              n273 = local read "shockOn_uS"() -> (w564:u32)
                              n274 = local read "timeout_uS"() -> (w563:u32)
                              n275 = local read "lickReward"() -> (w562:bool)
                              n276 = local read "toneReward"() -> (w561:bool)
                              n277 = local read "allowPunish"() -> (w560:bool)
                              n278 = local read "manualShock"() -> (w559:bool)
                              n279 = local read "manualWaterLeft"() -> (w558:bool)
                              n280 = local read "manualWaterRight"() -> (w557:bool)
                              n281 = local read "lickThreshold_V"() -> (w556:fxp<+/-,16,5>)
                              n282 = local read "vsThreshold_V"() -> (w555:fxp<+/-,16,5>)
                              n283 = local read "audioThreshold_V"() -> (w554:fxp<+/-,16,5>)
                              n284 = local read "audioOffState_V"() -> (w551:fxp<+/-,16,5>)
                              n285 = local read "audioFilterPeriod_uS"() -> (w553:i32)
                              n286 = local read "vsFilterPeriod_uS"() -> (w552:i32)
                              n287 = Build Array(w568, w567, w566, w565, w564, w563) -> (w550:u32[])
                              n288 = Build Array(w562, w561, w560, w559, w558, w557) -> (w539:bool[])
                              n289 = Boolean To (0,1)(Boolean=w539) -> (0, 1=w538:i16[])
                              n290 = Build Array(w556, w555, w554, w551, w553, w552) -> (w549:fxp<+/-,43,32>[])
                              n291 = Initialize Array(sgl 0.0, 2) -> (w546:sgl[])
                              n292 = Build Array (concatenate)(w550, w538, w549, w546) -> (w545:sgl[])
                              n293 = Array Size(array=w545) -> (size(s)=w541:i32)
                              n294 = Subtract(x=w545, y=w579) -> (x-y=w578:sgl[])
                              n295 = Reshape Array(w545, w541, 1 ("dimension size")) -> (w573:sgl[][])
                              n296 = Absolute Value(x=w578) -> (abs(x)=w576:sgl[])
                              n297 = Less?(x=w576, y=1e-06) -> (x < y?=w575:bool[])
                              n298 = Replace Array Subset(array=w574, new element=w573, index (row)=w543, index (col)=w542) -> (w572:sgl[][])
                              n299 = for {
                                tunnel: w575 -> [w601] mode=indexing
                                tunnel: w545 -> [w600] mode=indexing
                                shift-right: [w597] -> w571
                                shift-left: w544 -> [w598]
                                i -> [w599]
                                n300 = case shown="False" w601 {
                                tunnel: w600 -> [_ w610]
                                tunnel: w599 -> [_ w604]
                                tunnel: w598 -> [w602 w608]
                                tunnel: [w602 w607] -> w597
                                frame True {
                                }
                                frame False {
                                n301 = case shown="5" w604 {
                                tunnel: ["dly" "rwp" "rwf" "wdr" "shd" "tod" "lkr" "tlr" "alp" "msh" "mwl" "mwr" "lth" "vth" "ath" "aof" "afp" _ _ _] -> w603
                                frame 0, Default {
                                }
                                frame 1 {
                                }
                                frame 2 {
                                }
                                frame 3 {
                                }
                                frame 4 {
                                }
                                frame 5 {
                                }
                                frame 6 {
                                }
                                frame 7 {
                                }
                                frame 8 {
                                }
                                frame 9 {
                                }
                                frame 10 {
                                }
                                frame 11 {
                                }
                                frame 12 {
                                }
                                frame 13 {
                                }
                                frame 14 {
                                }
                                frame 15 {
                                }
                                frame 16 {
                                }
                                frame 17 {
                                (unwired) "vfp"
                                }
                                frame 18 {
                                }
                                frame 19 {
                                }
                                }
                                n302 = Format Value(format string="%.3f", value (0)=w610) -> (output string=w605:string)  [unwired: 1 in]
                                n303 = call <vilib>:"Space Constant.vi"() -> ("String"=w606:string)
                                n304 = Concatenate Strings(w608, w603, w606, w605, w606) -> (w607:string)
                                }
                                }
                              }
                              n305 = local read "VSmissed"() -> (w584:bool)
                              n306 = local read "stateMissed"() -> (w583:bool)
                              n307 = local read "CurTrial#"() -> (w587:u16)
                              n308 = local read "totalTrial#"() -> (w586:u16)
                              n309 = local read "run-stop"() -> (w582:bool)
                              n310 = Equal?(x=w587, y=w586) -> (x = y?=w585:bool)
                              n311 = Not(x=w582) -> (.not. x?=w580:bool)
                              n312 = Compound Arithmetic op=OR(w584, w583, w585) -> (w569:bool)
                              n313 = case shown="False" w569 {
                                frame False {
                                }
                                frame True {
                                n314 = local write "run-stop"(FALSE ("run-stop")) -> ()
                                }
                              }
                              n315 = Compound Arithmetic op=OR(w569, w580, w581) -> (w537:bool)
                              n316 = case shown="False" w537 {
                                tunnel: w571 -> [w592 _]
                                tunnel: [w588 w593] -> w570
                                frame False {
                                n317 = call <vilib>:"Space Constant.vi"() -> ("String"=w590:string)
                                n318 = Concatenate Strings(w592, "start" ("string"), w590, "1.000" ("string"), w590) -> (w588:string)
                                }
                                frame True {
                                n319 = call <vilib>:"Space Constant.vi"() -> ("String"=w595:string)
                                n320 = Concatenate Strings("stop" ("string"), w595, "1.000" ("string"), w595) -> (w593:string)
                                }
                              }
                            }
                            frame #2 {
                              n321 = local read "lickReward"() -> (w629:bool)
                              n322 = Or(x=w631, y=w629) -> (x .or. y?=w630:bool)
                              n323 = case shown="False" w630 {
                                tunnel: w633 -> [w634 w638]
                                tunnel: [w634 w637] -> w632
                                frame True {
                                }
                                frame False {
                                w636 = TRUE
                                n324 = Increment(x=w638) -> (x+1=w637:i32)
                                n325 = local write "CurTrial#"(w637) -> ()
                                n326 = local write "stateBusy"(w636) -> ()
                                n327 = local write "VSbusy"(w636) -> ()
                                n328 = local read "toneReward"() -> (w635:bool)
                                n329 = case shown="True" w635 {
                                frame False {
                                }
                                frame True {
                                n330 = disable-structure shown="Enabled" {
                                frame Enabled {
                                n331 = call "generateTone.vi"() -> ()  [unwired: 12 in]
                                }
                                frame Disabled {
                                }
                                }
                                n332 = local write "VSbusy"(FALSE) -> ()
                                }
                                }
                                }
                              }
                            }
                          }
                          n333 = local write "INFO"(w495) -> ()
                          n334 = local read "IP_broadcast"() -> (w496:string)
                          n335 = local read "port_remote"() -> (w494:u16)
                          n336 = String To IP(1:w496) -> (0:w497:u32)
                          n337 = UDP Write(address=w497, port or service name=w494, connection ID=w499, data in=w495, 8:w492) -> (error out=w493:errorcluster, 3:w498:refnum<k16>)  [unwired: 1 in]
                        }
                        frame True {
                          n338 = stacked-sequence {
                            seq-local: [w688 _] -> [_ w754]
                            seq-local: [w689 _] -> [_ w753]
                            tunnel: w651 -> [w700 _]
                            tunnel: w650 -> [w699 _]
                            tunnel: w649 -> [w695 _]
                            tunnel: [w655 _] -> w648
                            tunnel: [_ w748] -> w647
                            tunnel: [_ w750] -> w646
                            tunnel: w645 -> [_ w744]
                            tunnel: [_ w743] -> w644
                            tunnel: [w679 _] -> w643
                            tunnel: w640 -> [w652 _]
                            frame #0 {
                              # "beh para (20)"
                              n339 = local read "delay_uS"() -> (w678:u32)
                              n340 = local read "rewardPeriod_uS"() -> (w677:u32)
                              n341 = local read "rwdrefPeriod_uS"() -> (w676:u32)
                              n342 = local read "waterOn_uS"() -> (w675:u32)
                              n343 = local read "shockOn_uS"() -> (w674:u32)
                              n344 = local read "timeout_uS"() -> (w673:u32)
                              n345 = local read "lickReward"() -> (w672:bool)
                              n346 = local read "toneReward"() -> (w671:bool)
                              n347 = local read "allowPunish"() -> (w670:bool)
                              n348 = local read "manualShock"() -> (w669:bool)
                              n349 = local read "manualWaterLeft"() -> (w668:bool)
                              n350 = local read "manualWaterRight"() -> (w667:bool)
                              n351 = local read "lickThreshold_V"() -> (w666:fxp<+/-,16,5>)
                              n352 = local read "vsThreshold_V"() -> (w665:fxp<+/-,16,5>)
                              n353 = local read "audioThreshold_V"() -> (w664:fxp<+/-,16,5>)
                              n354 = local read "audioOffState_V"() -> (w661:fxp<+/-,16,5>)
                              n355 = local read "audioFilterPeriod_uS"() -> (w663:i32)
                              n356 = local read "vsFilterPeriod_uS"() -> (w662:i32)
                              n357 = Build Array(w678, w677, w676, w675, w674, w673) -> (w660:u32[])
                              n358 = Build Array(w672, w671, w670, w669, w668, w667) -> (w654:bool[])
                              n359 = Boolean To (0,1)(Boolean=w654) -> (0, 1=w653:i16[])
                              n360 = Build Array(w666, w665, w664, w661, w663, w662) -> (w659:fxp<+/-,43,32>[])
                              n361 = Initialize Array(sgl 0.0, 2) -> (w656:sgl[])
                              n362 = Build Array (concatenate)(w660, w653, w659, w656) -> (w655:sgl[])
                              n363 = Subtract(x=w655, y=w695) -> (x-y=w698:sgl[])
                              n364 = Absolute Value(x=w698) -> (abs(x)=w697:sgl[])
                              n365 = Less?(x=w697, y=1e-06) -> (x < y?=w694:bool[])
                              n366 = for {
                                tunnel: w694 -> [w703] mode=indexing
                                shift-right: [w704] -> w690
                                shift-left: "" -> [w705]
                                tunnel: w655 -> [w702] mode=indexing
                                i -> [w706]
                                n367 = case shown="False" w703 {
                                tunnel: w706 -> [w714 _]
                                tunnel: w705 -> [w710 w732]
                                tunnel: [w708 w732] -> w704
                                tunnel: w702 -> [w707 _]
                                frame False {
                                n368 = case shown="1" w714 {
                                tunnel: ["dly" "rwp" "rwf" "wdr" "shd" "tod" "lkr" "tlr" "alp" "msh" "mwl" "mwr" "lth" "vth" "ath" "aof" "afp" _ _ _] -> w709
                                frame 0, Default {
                                }
                                frame 1 {
                                }
                                frame 2 {
                                }
                                frame 3 {
                                }
                                frame 4 {
                                }
                                frame 5 {
                                }
                                frame 6 {
                                }
                                frame 7 {
                                }
                                frame 8 {
                                }
                                frame 9 {
                                }
                                frame 10 {
                                }
                                frame 11 {
                                }
                                frame 12 {
                                }
                                frame 13 {
                                }
                                frame 14 {
                                }
                                frame 15 {
                                }
                                frame 16 {
                                }
                                frame 17 {
                                (unwired) "vfp"
                                }
                                frame 18 {
                                }
                                frame 19 {
                                }
                                }
                                n369 = Format Value(format string="%.3f", value (0)=w707) -> (output string=w711:string)  [unwired: 1 in]
                                n370 = call <vilib>:"Space Constant.vi"() -> ("String"=w712:string)
                                n371 = Concatenate Strings(w710, w709, w712, w711, w712) -> (w708:string)
                                }
                                frame True {
                                }
                                }
                              }
                              n372 = String Length(string=w690) -> (length=w691:i32)
                              n373 = Not Equal To 0?(x=w691) -> (x != 0?=w692:bool)
                              n374 = case shown="False" w692 {
                                tunnel: w700 -> [w733 w742]
                                tunnel: w699 -> [w734 w741]
                                tunnel: w690 -> [_ w737]
                                tunnel: [w733 w736] -> w688
                                tunnel: [w734 w735] -> w689
                                frame False {
                                }
                                frame True {
                                n375 = local read "IP_broadcast"() -> (w739:string)
                                n376 = local read "port_remote"() -> (w738:u16)
                                n377 = String To IP(1:w739) -> (0:w740:u32)
                                n378 = UDP Write(address=w740, port or service name=w738, connection ID=w742, data in=w737, 8:w741) -> (error out=w735:errorcluster, 3:w736:refnum<k16>)  [unwired: 1 in]
                                }
                              }
                              n379 = local read "VSmissed"() -> (w683:bool)
                              n380 = local read "stateMissed"() -> (w684:bool)
                              n381 = local read "CurTrial#"() -> (w680:u16)
                              n382 = local read "totalTrial#"() -> (w681:u16)
                              n383 = local read "run-stop"() -> (w687:bool)
                              n384 = Equal?(x=w680, y=w681) -> (x = y?=w682:bool)
                              n385 = Not(x=w687) -> (.not. x?=w686:bool)
                              n386 = Compound Arithmetic op=OR(w683, w684, w682) -> (w685:bool)
                              n387 = case shown="True" w685 {
                                frame False {
                                }
                                frame True {
                                n388 = local write "run-stop"(FALSE ("run-stop")) -> ()
                                }
                              }
                              n389 = Compound Arithmetic op=OR(w685, w686, w652) -> (w679:bool)
                            }
                            frame #1 {
                              n390 = UDP Read(connection ID=w754, timeout ms (25000)=0, 8:w753) -> (data out=w745:string, error out=w752:errorcluster, 3:w748:refnum<k16>, 6:w746:u32)  [unwired: 1 in, 1 out]
                              n391 = String Length(string=w745) -> (length=w749:i32)
                              n392 = local write "Incoming data"(w745) -> ()
                              n393 = Not Equal To 0?(x=w749) -> (x != 0?=w747:bool)
                              n394 = case shown="True" w747 {
                                tunnel: w746 -> [_ w760]
                                tunnel: w745 -> [_ w766]
                                tunnel: w744 -> [w756 w759]
                                tunnel: [w756 w757] -> w743
                                frame False {
                                }
                                frame True {
                                n395 = Scan From String(format string="%s %f ", input string=w766, initial scan location=u32 0, default 1="no" ("default value 1"), default 2=-1.0 ("default value 2")) -> (output 1=w761:string, output 2=w758:dbl)  [unwired: 1 in, 3 out]
                                n396 = case shown="\"TrlDone\", Default" w761 {
                                tunnel: w760 -> [w779]
                                tunnel: w759 -> [w772]
                                tunnel: w758 -> [w773]
                                tunnel: [w772] -> w757
                                frame "TrlDone", Default {
                                n397 = Random Number (0-1)() -> (number: 0 to 1=w770:dbl)
                                n398 = local read "IP_RT"() -> (w777:string)
                                n399 = IP To String(1:TRUE ("dot notation? (F)"), 2:w779) -> (0:w774:string)
                                n400 = Multiply(x=w770, y="ITI_ms") -> (x*y=w767:dbl)
                                n401 = Match True/False String(2:"" ("false string"), 3:w777, 4:w774) -> (0:w775:bool)  [unwired: 1 out]
                                n402 = Add(x=3000, y=w767) -> (x+y=w768:dbl)
                                n403 = local write "Originating IP"(w774) -> ()
                                n404 = case shown="True" w775 {
                                tunnel: w774 -> [w785 _]
                                tunnel: w772 -> [w782 w799]
                                tunnel: w773 -> [w781 w800]
                                frame False {
                                n405 = local read "IP_VS"() -> (w784:string)
                                n406 = Match True/False String(2:"" ("false string"), 3:w784, 4:w785) -> (0:w780:bool)  [unwired: 1 out]
                                n407 = case shown="True" w780 {
                                tunnel: w782 -> [_ w792]
                                tunnel: w781 -> [_ w791]
                                frame False {
                                n408 = local write "Error 2"("Unknown source Error") -> ()
                                }
                                frame True {
                                n409 = Subtract(x=w791, y=w792) -> (x-y=w790:dbl)
                                n410 = Absolute Value(x=w790) -> (abs(x)=w789:dbl)
                                n411 = local write "VSbusy"(FALSE) -> ()
                                n412 = Greater?(x=w789, y=1e-06) -> (0:w787:bool)
                                n413 = local write "VSmissed"(w787) -> ()
                                }
                                }
                                }
                                frame True {
                                n414 = Subtract(x=w800, y=w799) -> (x-y=w798:dbl)
                                n415 = Absolute Value(x=w798) -> (abs(x)=w797:dbl)
                                n416 = Greater?(x=w797, y=1e-06) -> (0:w795:bool)
                                n417 = local write "stateBusy"(FALSE) -> ()
                                n418 = local write "stateMissed"(w795) -> ()
                                }
                                }
                                n419 = Wait (ms)(milliseconds to wait=w768) -> ()  [unwired: 1 out]
                                }
                                }
                                }
                              }
                              n420 = call "Remove_selected_error.vi"("error in (no error)"=w752, "errorCode"=56) -> ("error out"=w750:errorcluster)
                            }
                          }
                        }
                      }
                      n421 = local read "stop - local"() -> (w468:bool)
                      n422 = node-c288() -> ()  [unwired: 1 in, 1 out]
                    }
                    n423 = node-c288(w239) -> ()  [unwired: 1 out]
                    n424 = Release Queue(queue=w238, error in (no error)=w237) -> (error out=w226:errorcluster)  [unwired: 1 in, 2 out]
                    n425 = To Single Precision Float(number=w252) -> (single precision float=w254:sgl[][])
                    n426 = local read "Save data"() -> (w253:bool)
                    n427 = case shown="True" w253 {
                      tunnel: w233 -> [w453 w467]
                      tunnel: w234 -> [_ w466]
                      tunnel: w254 -> [_ w457]
                      tunnel: [w453 w454] -> w225
                      frame False {
                      }
                      frame True {
                        n428 = Multiply(x=502, y=4) -> (x*y=w462:i32)
                        n429 = Set File Position(offset (in bytes) (0)=w462, refnum=w466, from (0:start)=enum16{"start", "end", "current"}."start", error in=w467) -> (refnum out=w459:refnum<file>, error out=w460:errorcluster)
                        n430 = Write to Binary File(file (use dialog)=w459, data=w457, error in=w460, 5:FALSE ("prepend array or string size? (T)"), 9:T3."little-endian" ("byte order (0:big-endian, network order)")) -> (refnum out=w455:refnum<file>, error out=w456:errorcluster)  [unwired: 1 in, 1 out]
                        n431 = Close File(refnum=w455, error in=w456) -> (error out=w454:errorcluster)  [unwired: 1 out]
                      }
                    }
                    n432 = node-c288(w241) -> ()  [unwired: 1 out]
                    n433 = node-c288(w275) -> ()  [unwired: 1 out]
                    n434 = Release Queue(queue=w232, error in (no error)=w231) -> (error out=w227:errorcluster)  [unwired: 1 in, 2 out]
                    n435 = Destroy Stream Endpoint(8:w268, 11:w271) -> (0:w229:errorcluster)
                    n436 = flat-sequence {
                      tunnel: w223 -> [w314]
                      frame #0 {
                        n437 = call <vilib>:"Simple Error Handler.vi"("error in (no error)"=w314) -> ()  [unwired: 4 in, 5 out]
                        n438 = shared-variable "Sabrina-RT1\\variables - network - RT (separate).lvlib\\stop - network"(FALSE ("stop - network")) -> ()  [unwired: 1 in, 1 out]
                      }
                    }
                    n439 = node-c288(w266) -> ()  [unwired: 1 out]
                    n440 = UDP Close(connection ID=w260, 8:w259) -> (error out=w230:errorcluster)  [unwired: 1 out]
                    n441 = Merge Errors(w230, w229, w224, w228, w227, w226, w225) -> (w223:errorcluster)
                  }
                }
              }
              frame 2 {
                n442 = local read "IP_host"() -> (w871:string)
                n443 = local read "port_local"() -> (w872:u16)
                n444 = String To IP(1:w871) -> (0:w870:u32)
                n445 = UDP Open(7:w870, 11:w872) -> (port=w874:refnum<k16>, 0:w875:errorcluster)  [unwired: 3 in, 1 out]
                n446 = local read "IP_broadcast"() -> (w868:string)
                n447 = local read "port_remote"() -> (w869:u16)
                n448 = String To IP(1:w868) -> (0:w873:u32)
                n449 = UDP Write(address=w873, port or service name=w869, connection ID=w874, data in="exit 1.000 ", 8:w875) -> (error out=w877:errorcluster, 3:w876:refnum<k16>)  [unwired: 1 in]
                n450 = UDP Close(connection ID=w876, 8:w877) -> (error out=w878:errorcluster)  [unwired: 1 out]
                n451 = call <vilib>:"Simple Error Handler.vi"("error in (no error)"=w878) -> ()  [unwired: 4 in, 5 out]
              }
            }
          }
          frame #2 {
            n452 = Wait (ms)(milliseconds to wait=u32 5) -> ()  [unwired: 1 out]
          }
        }
      }
    }
  }
